vi "Gather_Deal_Data.vi"(8 "strModelChoice":string(combo)="WW6500", 10 "1号机端口":refnum<visa-resource-name>="COM1") -> (2 "缓冲区数据":u32=278, 3 "strResultArrayOut":string[](array[string])=["WaterLevel:22751", "WaterTemp:287", "AirTemp:300", "IPMTemp:300", "MotorActualRPM:0", "MotorTargetRPM:0", "FanActualRPM:0", "MemsSensorA:0", "MemsSensorB:35", "MemsSensorC:0", "WaterThermistorADC:33242", "TouchSensor:0", "LeakageSensor:0", "DCLink:321", "IsDoorOpen:0", "IsTimeShort:0", "Progress:0", "Step:0", "TotalRemainTime:3240", "StepRemainTime:0", "WeightSensingLowData:240", "WeightSensingResult:240", "ColdValve:0", "HotValve:0", "PreValve:0", "WaterShotValve:0", "BleachValve:0", "DryValve:0", "SteamValve:0", "SoftenerValve:0", "FilterValve:0", "IsDoorLocked:1", "SSRCommon:0", "MainRelay:1", "ACTUATOR2:0", "WaterDrainer:0", "CirculationPump:0", "WaterHeater:0", "DryHeater:0", "SteamHeater:0", "MotorDriveDirection:1", "IsDoubleDoorOpen:0", "IsDoubleDoorLock:1", "RunStateID:0", "PowerStateID:5", "SoundID:241", "ErrorCode:32323232", "OptionData:4112", "MainVersion:114494850", "SUBVersion:110484951", "InverterVersion:57484866", "MainVersion:32324853"], 9 "写指令":bool)   [LabVIEW 2011]
uses:
  <vilib>/Instr/_visa.llb/VISA Configure Serial Port (Instr).vi
  GlobalVariable/strGlobalVariable.vi
panel:
  out "mu083rdCmdSendCount":u8
  out "mu08SendCountStop":u8=9
  out "mbfSendStop":bool=TRUE
  out "WWorWD":bool
  out "1st_OnorOff":bool
  in  "chart":bool
  in  "Start":bool=TRUE
  out "mu08BufSize":u8=139
  out "mbfDealData":bool=TRUE
  in  "mu08SendCmd":u8=4
  in  "CmdNumCount":u8=76
  out "mu08ArrayBuf0":u8[](array[numeric])=[44, 7, 1, 44, 11, 0, 0, 12, 0, 0, 13, 0, 0, 21, 0, 0, 22, 0, 35, 23, 0, 0, 24, 129, 218, 29, 0, 0, 0, 0, 31, 0, 0, 33, 0, 34, 1, 65, 35, 0, 41, 0, 42, 0, 43, 0, 44, 12, 168, 45, 0, 0, 46, 0, 240, 47, 240, 48, 0, 49, 0, 50, 136, 51, 0, 52, 0, 53, 0, 54, 132, 58, 0, 59, 5, 60, 241, 61, 32, 32, 32, 32, 82, 4, 112, 83, 90, 3, 4, 0, 2, 4, 0, 0, 0, 0, 2, 0, 0, 0, 105, 201, 114, 49, 48, 50, 202, 110, 48, 49, 51, 203, 57, 48, 48, 66, 204, 32, 32, 48, 53, 251, 6, 239, 78, 90, 165, 139, 1, 240, 0, 1, 88, 223, 2, 1, 31, 3, 1, 44, 7, 1, 44, 11, 0, 0, 12, 0, 0, 13, 0, 0, 21, 0, 0, 22, 0, 35, 23, 0, 0, 24, 129, 218, 29, 0, 0, 0, 0, 31, 0, 0, 33, 0, 34, 1, 65, 35, 0, 41, 0, 42, 0, 43, 0, 44, 12, 168, 45, 0, 0, 46, 0, 240, 47, 240, 48, 0, 49, 0, 50, 136, 51, 0, 52, 0, 53, 0, 54, 132, 58, 0, 59, 5, 60, 241, 61, 32, 32, 32, 32, 82, 4, 112, 83, 90, 3, 4, 0, 2, 4, 0, 0, 0, 0, 2, 0, 0, 0, 105, 201, 114, 49, 48, 50, 202, 110, 48, 49, 51, 203, 57, 48, 48, 66, 204, 32, 32, 48, 53, 251, 6, 239, 78, 90, 165, 139, 1, 240, 0, 1, 88, 217, 2, 1, 31, 3, 1] format="0x%x"
  out "mu16ArrayBuf0":u16=278
  out "mu08ArrayDatas":u8[](array[numeric])=[90, 165, 139, 1, 240, 0, 1, 88, 223, 2, 1, 31, 3, 1, 44, 7, 1, 44, 11, 0, 0, 12, 0, 0, 13, 0, 0, 21, 0, 0, 22, 0, 35, 23, 0, 0, 24, 129, 218, 29, 0, 0, 0, 0, 31, 0, 0, 33, 0, 34, 1, 65, 35, 0, 41, 0, 42, 0, 43, 0, 44, 12, 168, 45, 0, 0, 46, 0, 240, 47, 240, 48, 0, 49, 0, 50, 136, 51, 0, 52, 0, 53, 0, 54, 132, 58, 0, 59, 5, 60, 241, 61, 32, 32, 32, 32, 82, 4, 112, 83, 90, 3, 4, 0, 2, 4, 0, 0, 0, 0, 2, 0, 0, 0, 105, 201, 114, 49, 48, 50, 202, 110, 48, 49, 51, 203, 57, 48, 48, 66, 204, 32, 32, 48, 53, 251, 6, 239, 78] format="0x%x"
  out "mu08ArrayDatasSize":u16=139
  out "命令":string
  in  "mbfUartClearOne":bool=TRUE
  out "Time":u32=400
  out "2nd_OnOrOff":bool
  in  "chart_2":bool
  in  "Start_2":bool
  in  "CmdNumCount 2":u8
  out "strResultArrayOut 2":string[](array[string])
  out "mbfDealData 2":bool
  out "mu08SendCmd_2":u8
  in  "写指令_2":bool=TRUE
  out "Time_2":u32=400
  out "缓冲区数据_2":u32=284
  out "mu08ArrayBuf0 2":u8[](array[numeric])=[90, 165, 142, 1, 240, 0, 1, 88, 200, 2, 0, 207, 3, 0, 219, 7, 1, 40, 11, 0, 0, 12, 0, 0, 13, 0, 0, 14, 0, 0, 21, 0, 0, 22, 0, 0, 23, 0, 0, 24, 150, 154, 29, 0, 0, 0, 0, 31, 0, 0, 33, 0, 34, 1, 64, 35, 0, 41, 0, 42, 0, 43, 0, 44, 12, 158, 45, 0, 0, 46, 0, 240, 47, 240, 48, 0, 49, 0, 50, 136, 51, 0, 52, 0, 53, 0, 54, 132, 58, 0, 59, 0, 60, 241, 61, 32, 32, 32, 32, 82, 64, 73, 83, 90, 2, 4, 0, 2, 4, 0, 0, 0, 0, 2, 0, 0, 0, 104, 201, 113, 49, 49, 53, 202, 70, 52, 48, 53, 203, 57, 48, 48, 66, 204, 32, 32, 48, 53, 251, 6, 87, 112, 90, 165, 142, 1, 240, 0, 1, 88, 200, 2, 0, 207, 3, 0, 219, 7, 1, 40, 11, 0, 0, 12, 0, 0, 13, 0, 0, 14, 0, 0, 21, 0, 0, 22, 0, 0, 23, 0, 0, 24, 150, 151, 29, 0, 0, 0, 0, 31, 0, 0, 33, 0, 34, 1, 64, 35, 0, 41, 0, 42, 0, 43, 0, 44, 12, 158, 45, 0, 0, 46, 0, 240, 47, 240, 48, 0, 49, 0, 50, 136, 51, 0, 52, 0, 53, 0, 54, 132, 58, 0, 59, 0, 60, 241, 61, 32, 32, 32, 32, 82, 64, 73, 83, 90, 2, 4, 0, 2, 4, 0, 0, 0, 0, 2, 0, 0, 0, 104, 201, 113, 49, 49, 53, 202, 70, 52, 48, 53, 203, 57, 48, 48, 66, 204, 32, 32, 48, 53, 251, 6, 95, 118] format="0x%x"
  out "mu16ArrayBuf0_2":u16=284
  out "mu08ArrayDatas_2":u8[](array[numeric])=[90, 165, 142, 1, 240, 0, 1, 88, 200, 2, 0, 207, 3, 0, 219, 7, 1, 40, 11, 0, 0, 12, 0, 0, 13, 0, 0, 14, 0, 0, 21, 0, 0, 22, 0, 0, 23, 0, 0, 24, 150, 154, 29, 0, 0, 0, 0, 31, 0, 0, 33, 0, 34, 1, 64, 35, 0, 41, 0, 42, 0, 43, 0, 44, 12, 158, 45, 0, 0, 46, 0, 240, 47, 240, 48, 0, 49, 0, 50, 136, 51, 0, 52, 0, 53, 0, 54, 132, 58, 0, 59, 0, 60, 241, 61, 32, 32, 32, 32, 82, 64, 73, 83, 90, 2, 4, 0, 2, 4, 0, 0, 0, 0, 2, 0, 0, 0, 104, 201, 113, 49, 49, 53, 202, 70, 52, 48, 53, 203, 57, 48, 48, 66, 204, 32, 32, 48, 53, 251, 6, 87, 112] format="0x%x"
  out "mu08ArrayDatasSize_2":u16=142
  out "mu08BufSize_2":u8
  in  "strModelChoice_2":string(combo)="WD5500"
  out "命令_2":string
  in  "mbfUartClearOne 2":bool=TRUE
  in  "2号机端口":refnum<visa-resource-name>="COM3"
  out "3rd_OnorOff":bool
  in  "chart_3":bool
  in  "Start_3":bool
  out "命令_3":string
  in  "CmdNumCount_3":u8
  out "mu16ArrayBuf0_3":u16=284
  out "mu08ArrayDatasSize_3":u16=142
  out "mu08BufSize_3":u8
  out "mu08ArrayBuf0_3":u8[](array[numeric])=[90, 165, 142, 1, 240, 0, 1, 88, 200, 2, 0, 207, 3, 0, 219, 7, 1, 40, 11, 0, 0, 12, 0, 0, 13, 0, 0, 14, 0, 0, 21, 0, 0, 22, 0, 0, 23, 0, 0, 24, 150, 154, 29, 0, 0, 0, 0, 31, 0, 0, 33, 0, 34, 1, 64, 35, 0, 41, 0, 42, 0, 43, 0, 44, 12, 158, 45, 0, 0, 46, 0, 240, 47, 240, 48, 0, 49, 0, 50, 136, 51, 0, 52, 0, 53, 0, 54, 132, 58, 0, 59, 0, 60, 241, 61, 32, 32, 32, 32, 82, 64, 73, 83, 90, 2, 4, 0, 2, 4, 0, 0, 0, 0, 2, 0, 0, 0, 104, 201, 113, 49, 49, 53, 202, 70, 52, 48, 53, 203, 57, 48, 48, 66, 204, 32, 32, 48, 53, 251, 6, 87, 112, 90, 165, 142, 1, 240, 0, 1, 88, 200, 2, 0, 207, 3, 0, 219, 7, 1, 40, 11, 0, 0, 12, 0, 0, 13, 0, 0, 14, 0, 0, 21, 0, 0, 22, 0, 0, 23, 0, 0, 24, 150, 151, 29, 0, 0, 0, 0, 31, 0, 0, 33, 0, 34, 1, 64, 35, 0, 41, 0, 42, 0, 43, 0, 44, 12, 158, 45, 0, 0, 46, 0, 240, 47, 240, 48, 0, 49, 0, 50, 136, 51, 0, 52, 0, 53, 0, 54, 132, 58, 0, 59, 0, 60, 241, 61, 32, 32, 32, 32, 82, 64, 73, 83, 90, 2, 4, 0, 2, 4, 0, 0, 0, 0, 2, 0, 0, 0, 104, 201, 113, 49, 49, 53, 202, 70, 52, 48, 53, 203, 57, 48, 48, 66, 204, 32, 32, 48, 53, 251, 6, 95, 118] format="0x%x"
  out "缓冲区数据_3":u32=284
  out "mu08ArrayDatas_3":u8[](array[numeric])=[90, 165, 142, 1, 240, 0, 1, 88, 200, 2, 0, 207, 3, 0, 219, 7, 1, 40, 11, 0, 0, 12, 0, 0, 13, 0, 0, 14, 0, 0, 21, 0, 0, 22, 0, 0, 23, 0, 0, 24, 150, 154, 29, 0, 0, 0, 0, 31, 0, 0, 33, 0, 34, 1, 64, 35, 0, 41, 0, 42, 0, 43, 0, 44, 12, 158, 45, 0, 0, 46, 0, 240, 47, 240, 48, 0, 49, 0, 50, 136, 51, 0, 52, 0, 53, 0, 54, 132, 58, 0, 59, 0, 60, 241, 61, 32, 32, 32, 32, 82, 64, 73, 83, 90, 2, 4, 0, 2, 4, 0, 0, 0, 0, 2, 0, 0, 0, 104, 201, 113, 49, 49, 53, 202, 70, 52, 48, 53, 203, 57, 48, 48, 66, 204, 32, 32, 48, 53, 251, 6, 87, 112] format="0x%x"
  in  "strModelChoice 2":string(combo)="WD5500"
  in  "写指令_3":bool=TRUE
  in  "3号机端口":refnum<visa-resource-name>="COM3"
  in  "mbfUartClearOne_3":bool=TRUE
  out "mbfDealData_3":bool
  out "Time_3":u32=400
  out "strResultArrayOut_3":string[](array[string])
  out "mu08SendCmd_2 2":u8
  out "4ed_OronOff":bool
  in  "chart_4":bool
  in  "Start_4":bool
  in  "strModelChoice_4":string(combo)="WD5500"
  out "Time_4":u32=400
  out "mbfDealData_4":bool
  in  "mbfUartClearOne_4":bool=TRUE
  out "strResultArrayOut_4":string[](array[string])
  out "mu08SendCmd_4":u8
  out "命令_4":string
  in  "写指令_4":bool=TRUE
  out "mu08ArrayDatas_4":u8[](array[numeric])=[90, 165, 142, 1, 240, 0, 1, 88, 200, 2, 0, 207, 3, 0, 219, 7, 1, 40, 11, 0, 0, 12, 0, 0, 13, 0, 0, 14, 0, 0, 21, 0, 0, 22, 0, 0, 23, 0, 0, 24, 150, 154, 29, 0, 0, 0, 0, 31, 0, 0, 33, 0, 34, 1, 64, 35, 0, 41, 0, 42, 0, 43, 0, 44, 12, 158, 45, 0, 0, 46, 0, 240, 47, 240, 48, 0, 49, 0, 50, 136, 51, 0, 52, 0, 53, 0, 54, 132, 58, 0, 59, 0, 60, 241, 61, 32, 32, 32, 32, 82, 64, 73, 83, 90, 2, 4, 0, 2, 4, 0, 0, 0, 0, 2, 0, 0, 0, 104, 201, 113, 49, 49, 53, 202, 70, 52, 48, 53, 203, 57, 48, 48, 66, 204, 32, 32, 48, 53, 251, 6, 87, 112] format="0x%x"
  in  "CmdNumCount_4":u8
  out "缓冲区数据_4":u32=284
  out "mu08BufSize_4":u8
  out "mu08ArrayBuf0_4":u8[](array[numeric])=[90, 165, 142, 1, 240, 0, 1, 88, 200, 2, 0, 207, 3, 0, 219, 7, 1, 40, 11, 0, 0, 12, 0, 0, 13, 0, 0, 14, 0, 0, 21, 0, 0, 22, 0, 0, 23, 0, 0, 24, 150, 154, 29, 0, 0, 0, 0, 31, 0, 0, 33, 0, 34, 1, 64, 35, 0, 41, 0, 42, 0, 43, 0, 44, 12, 158, 45, 0, 0, 46, 0, 240, 47, 240, 48, 0, 49, 0, 50, 136, 51, 0, 52, 0, 53, 0, 54, 132, 58, 0, 59, 0, 60, 241, 61, 32, 32, 32, 32, 82, 64, 73, 83, 90, 2, 4, 0, 2, 4, 0, 0, 0, 0, 2, 0, 0, 0, 104, 201, 113, 49, 49, 53, 202, 70, 52, 48, 53, 203, 57, 48, 48, 66, 204, 32, 32, 48, 53, 251, 6, 87, 112, 90, 165, 142, 1, 240, 0, 1, 88, 200, 2, 0, 207, 3, 0, 219, 7, 1, 40, 11, 0, 0, 12, 0, 0, 13, 0, 0, 14, 0, 0, 21, 0, 0, 22, 0, 0, 23, 0, 0, 24, 150, 151, 29, 0, 0, 0, 0, 31, 0, 0, 33, 0, 34, 1, 64, 35, 0, 41, 0, 42, 0, 43, 0, 44, 12, 158, 45, 0, 0, 46, 0, 240, 47, 240, 48, 0, 49, 0, 50, 136, 51, 0, 52, 0, 53, 0, 54, 132, 58, 0, 59, 0, 60, 241, 61, 32, 32, 32, 32, 82, 64, 73, 83, 90, 2, 4, 0, 2, 4, 0, 0, 0, 0, 2, 0, 0, 0, 104, 201, 113, 49, 49, 53, 202, 70, 52, 48, 53, 203, 57, 48, 48, 66, 204, 32, 32, 48, 53, 251, 6, 95, 118] format="0x%x"
  in  "4号机端口":refnum<visa-resource-name>="COM3"
  out "mu08ArrayDatasSize_4":u16=142
  out "mu16ArrayBuf0_4":u16=284
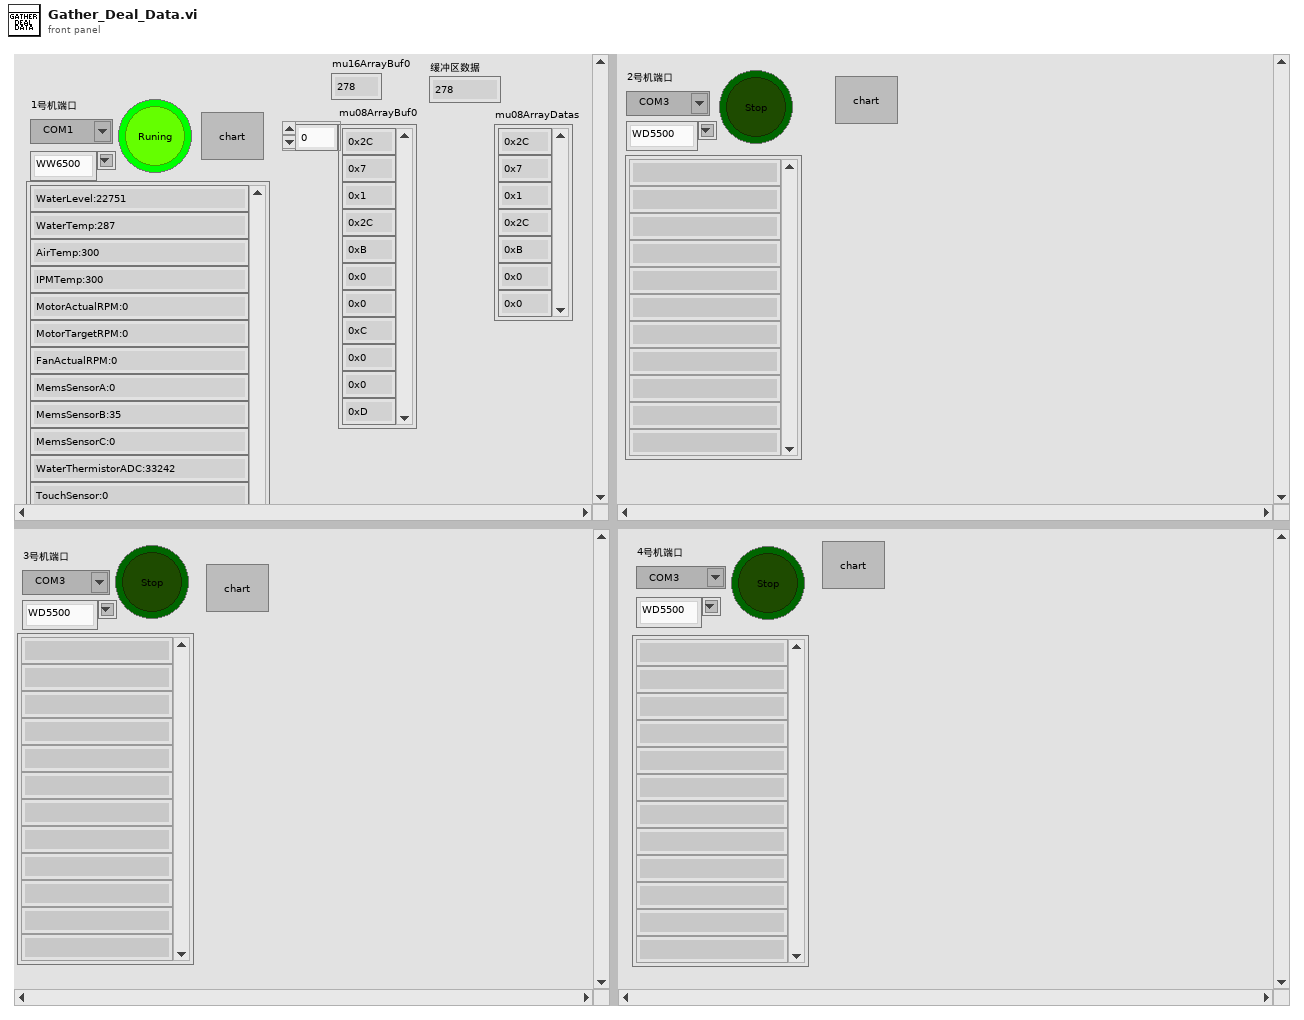
[diagram p1: front panel]
types:
  T1 = enum16{"open", "replace", "create", "open or create", "replace or create", "replace or create with confirmation"}
  T2 = enum32{"Invalid", "Standard", "Closed", "Hidden", "Minimized", "Maximized"}
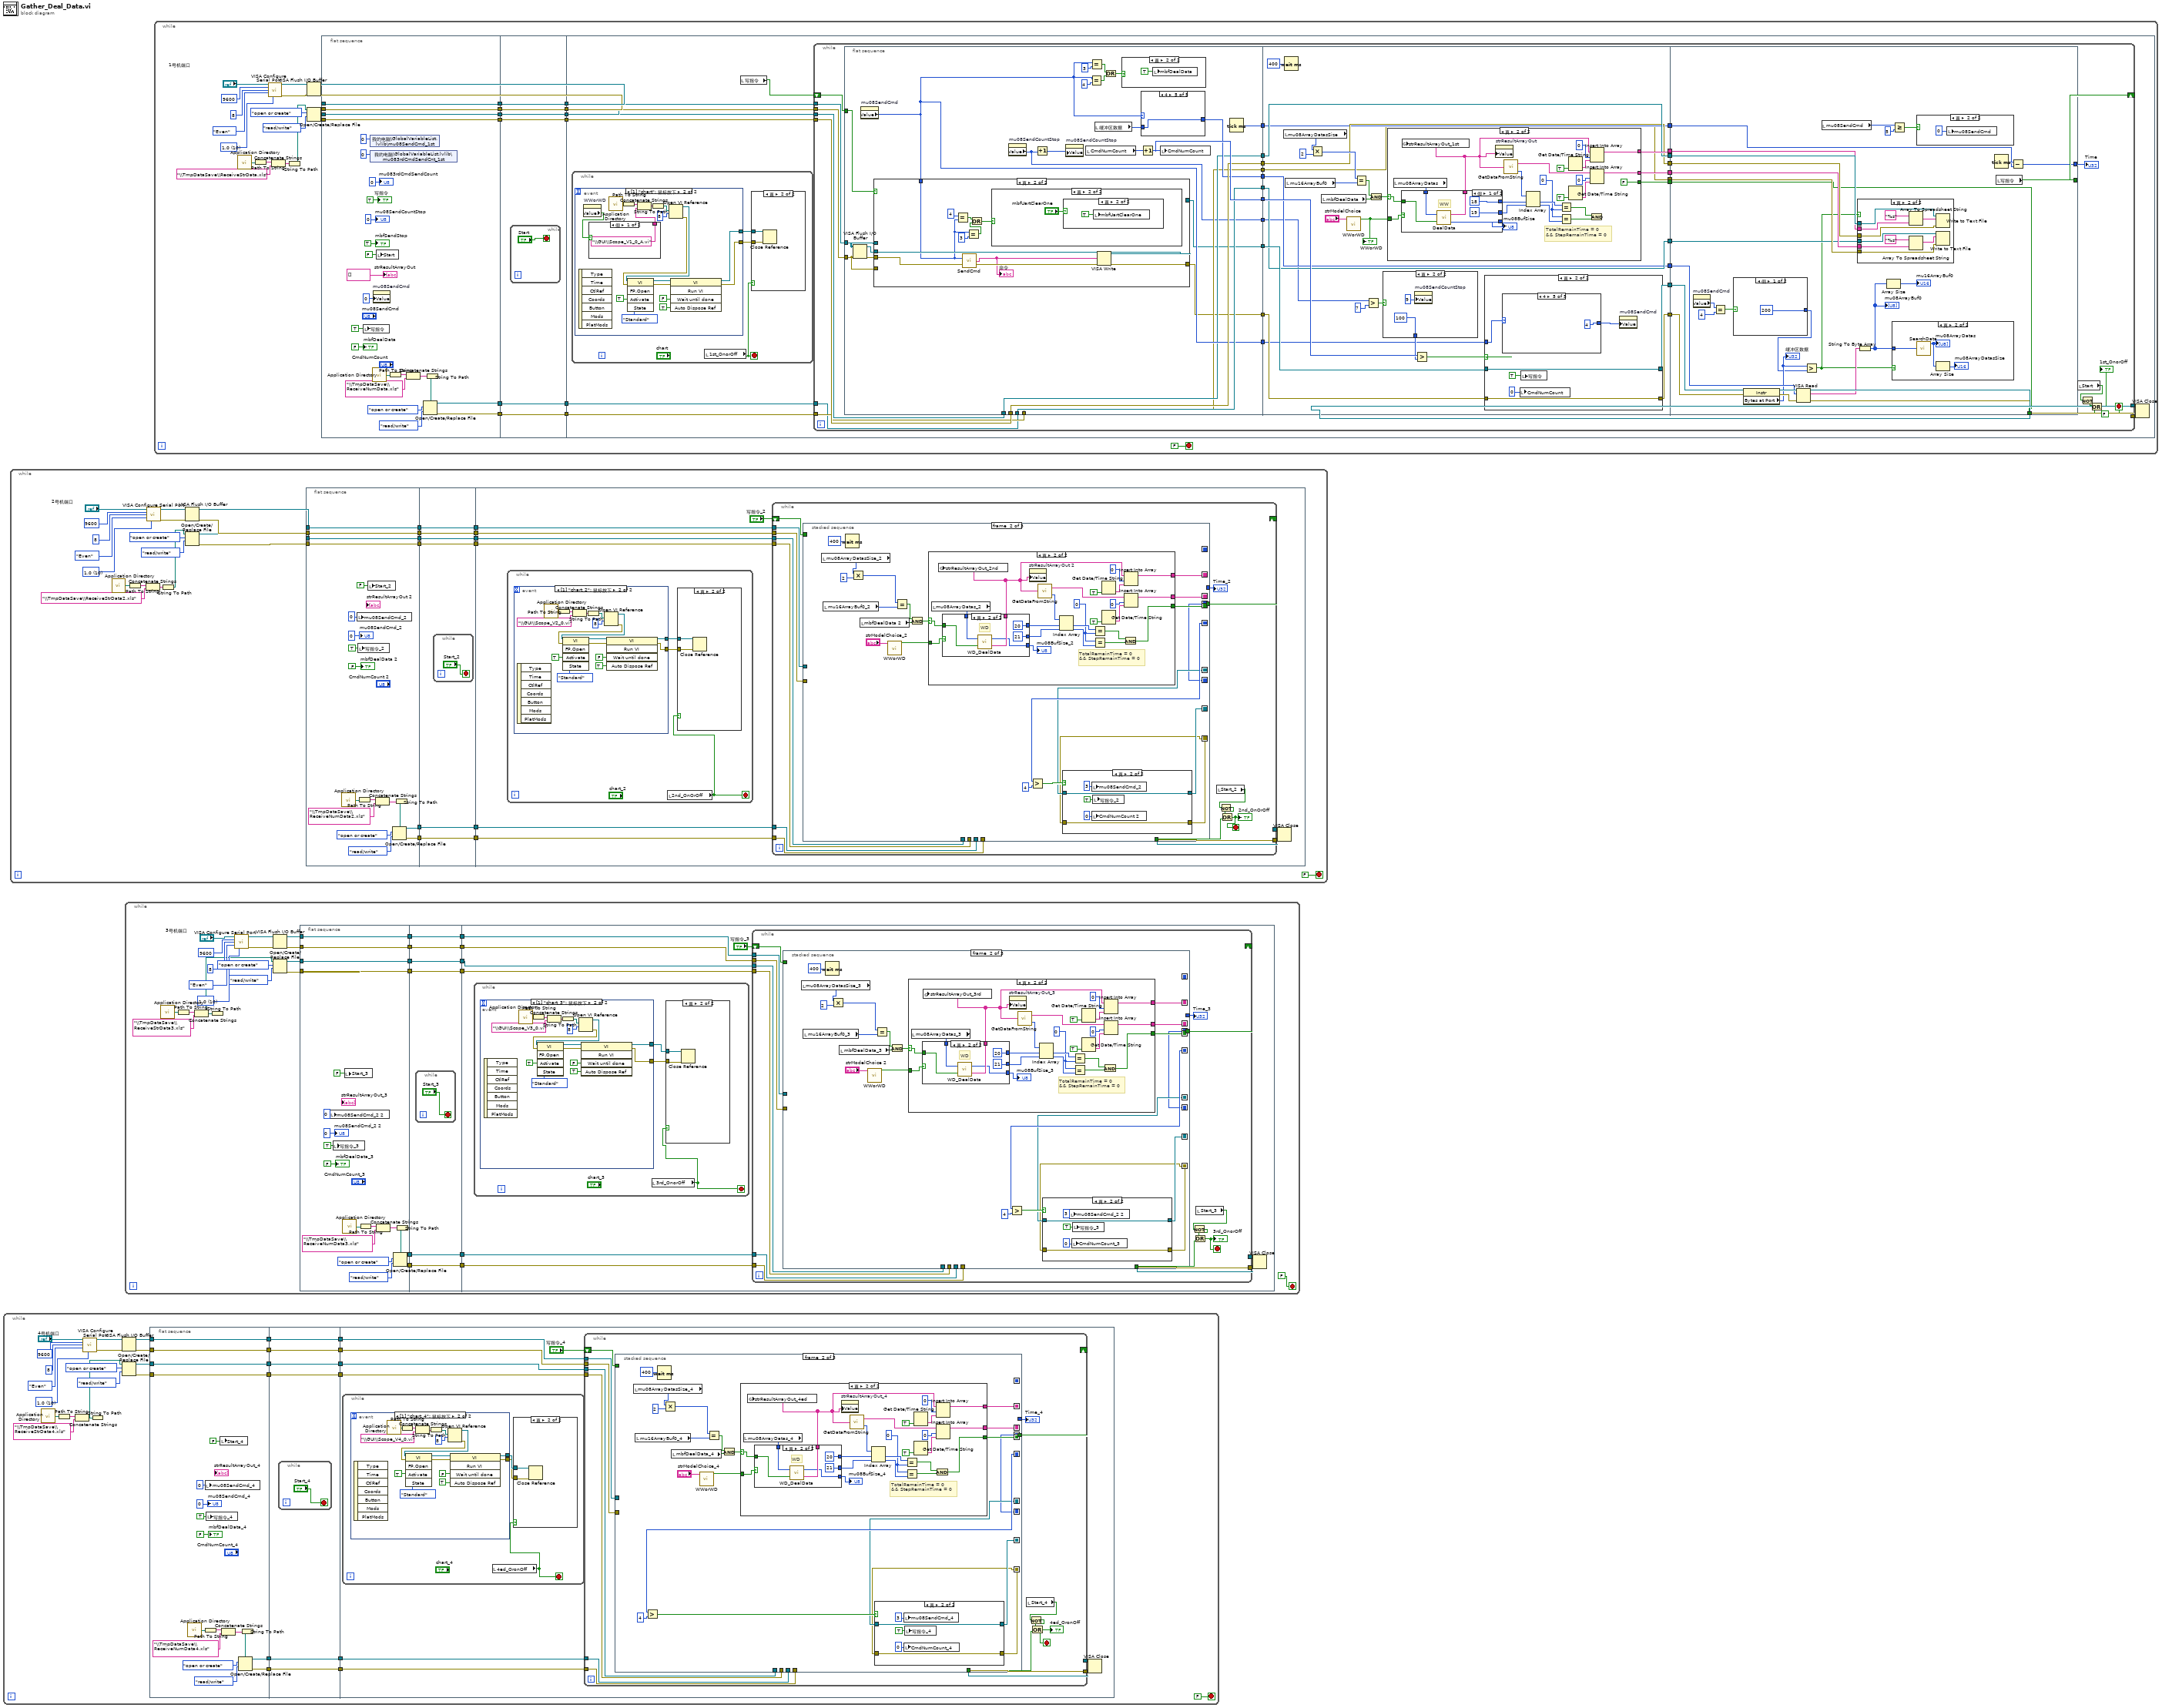
[diagram p0: block diagram]
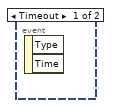
[diagram p3: hidden frame]
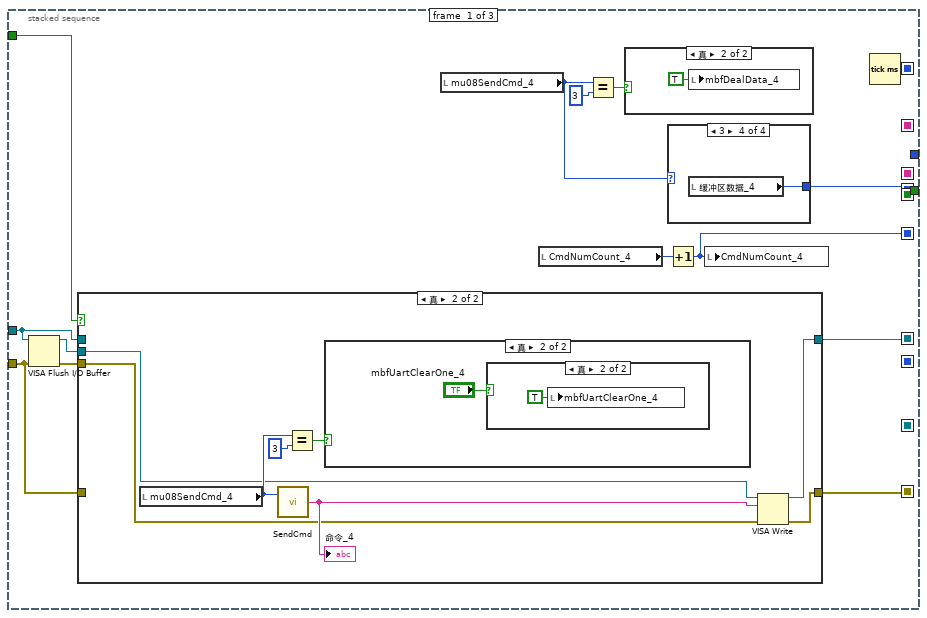
[diagram p4: hidden frame]
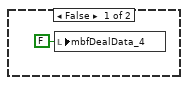
[diagram p5: hidden frame]
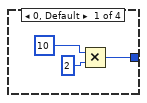
[diagram p6: hidden frame]
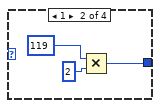
[diagram p7: hidden frame]
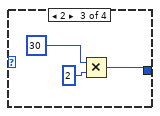
[diagram p8: hidden frame]
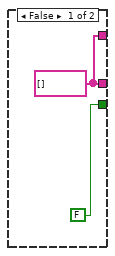
[diagram p12: hidden frame]
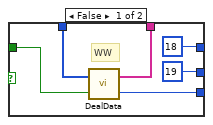
[diagram p13: hidden frame]
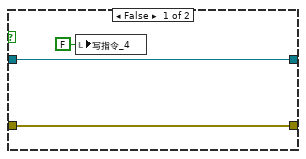
[diagram p14: hidden frame]
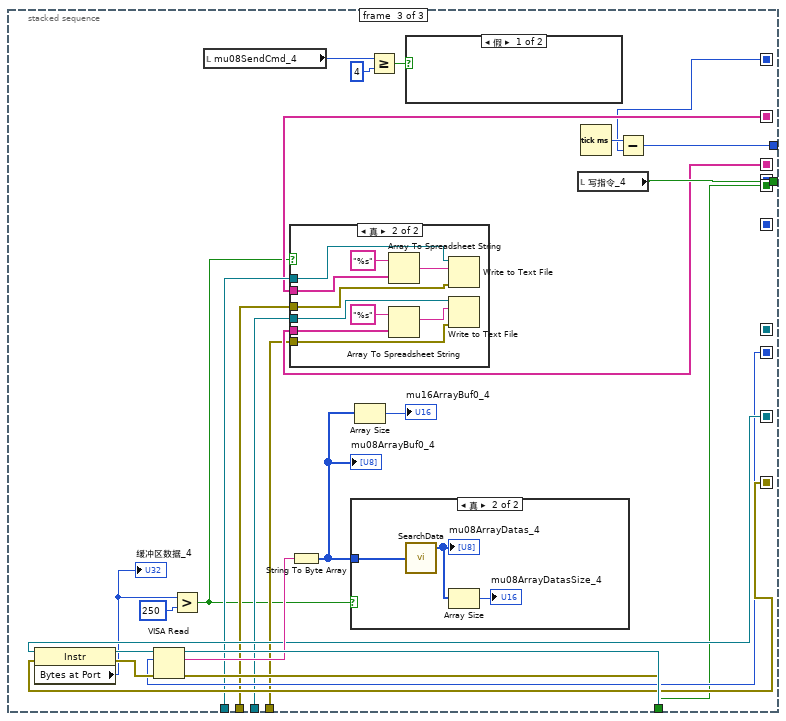
[diagram p15: hidden frame]
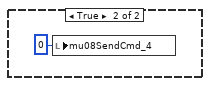
[diagram p18: hidden frame]
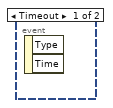
[diagram p20: hidden frame]
diagram:
  n1 = while {
    stop <- FALSE stop-if-true
    w15 = u16 10 items=["1.0"=10, "1.5"=15, "2.0"=20] ("stop bits (10: 1 bit)")
    n2 = call <vilib>:"Application Directory.vi"() -> ("Application Directory"=w5:path)
    n3 = Path To String(path=w5) -> (string=w4:string)
    n4 = Concatenate Strings(w4, "\\TmpDataSave\\ReceiveStrData4.xls" ("字符串")) -> (w2:string)
    n5 = call-poly "VISA Configure Serial Port"("VISA resource name"="4号机端口", "baud rate (9600)"=u32 9600, "data bits (8)"=u16 8, "parity (0:none)"=enum16{"None", "Odd", "Even", "Mark", "Space"}."Even", "stop bits (10: 1 bit)"=w15) -> ("VISA resource name out"=w14:refnum<visa-resource-name>, "error out"=w13:errorcluster)  [unwired: 9 in]
    n6 = String To Path(string=w2) -> (path=w8:path)
    n7 = VISA Flush I/O Buffer(VISA resource name=w14, error in (no error)=w13) -> (VISA resource name out=w12:refnum<visa-resource-name>, error out=w11:errorcluster)  [unwired: 1 in]
    n8 = Open/Create/Replace File(file path (use dialog)=w8, operation (0:open)=T1."open or create" ("操作(0:open)"), access (0:read/write)=enum16{"read/write", "read-only", "write-only"}."read/write" ("权限(0:read/write)")) -> (refnum out=w7:refnum<file>, error out=w6:errorcluster)  [unwired: 3 in, 1 out]
    n9 = flat-sequence {
      tunnel: w6 -> [w46]
      tunnel: w7 -> [w47]
      tunnel: w11 -> [w48]
      tunnel: w12 -> [w49]
      tunnel: [w49] -> w31
      tunnel: [w48] -> w30
      tunnel: [w47] -> w29
      tunnel: [w46] -> w28
      tunnel: [w32] -> w27
      tunnel: [w33] -> w26
      tunnel: [w55] -> w25
      tunnel: [w54] -> w24
      tunnel: [w53] -> w23
      tunnel: [w52] -> w22
      tunnel: [w51] -> w21
      tunnel: [w50] -> w20
      tunnel: w31 -> [w55]
      tunnel: w30 -> [w54]
      tunnel: w29 -> [w53]
      tunnel: w28 -> [w52]
      tunnel: w27 -> [w51]
      tunnel: w26 -> [w50]
      tunnel: w25 -> [w62]
      tunnel: w24 -> [w61]
      tunnel: w23 -> [w60]
      tunnel: w22 -> [w59]
      tunnel: w21 -> [w58]
      tunnel: w20 -> [w57]
      frame #0 {
        n10 = call <vilib>:"Application Directory.vi"() -> ("Application Directory"=w37:path)
        n11 = Path To String(path=w37) -> (string=w38:string)
        n12 = local write "mu08SendCmd_4"(u8 0 ("Cmd值")) -> ()
        n13 = local write "写指令_4"(TRUE ("写指令")) -> ()
        n14 = local write "Start_4"(FALSE ("Start_4")) -> ()
        n15 = Concatenate Strings(w38, "\\TmpDataSave\\ReceiveNumData4.xls" ("字符串")) -> (w40:string)
        n16 = String To Path(string=w40) -> (path=w36:path)
        n17 = Open/Create/Replace File(file path (use dialog)=w36, operation (0:open)=T1."open or create" ("操作(0:open)"), access (0:read/write)=enum16{"read/write", "read-only", "write-only"}."read/write" ("权限(0:read/write)")) -> (refnum out=w33:refnum<file>, error out=w32:errorcluster)  [unwired: 3 in, 1 out]
        "mu08SendCmd_4" <- u8 0 ("mu08SendCmd")
        "mbfDealData_4" <- FALSE ("mbfDealData")
      }
      frame #1 {
        n18 = while {
          stop <- "Start_4" stop-if-true
        }
      }
      frame #2 {
        n19 = while {
          stop <- w67 stop-if-true
          n20 = event shown="[1] \"chart_4\": 鼠标按下" {
            selector: _ -> [_ _]
            dyn-events: _ -> [_ _]
            timeout: _ -> [_ _]
            tunnel: [_ w72] -> w68
            tunnel: [_ w71] -> w66
            event Timeout {
              n21 = event-data() -> ()  [unwired: 1 in, 2 out]
            }
            event "chart_4": Mouse Down {
              n22 = event-data() -> ()  [unwired: 1 in, 7 out]
              n23 = call <vilib>:"Application Directory.vi"() -> ("Application Directory"=w84:path)
              n24 = Path To String(path=w84) -> (string=w83:string)
              n25 = Concatenate Strings(w83, "\\GUI\\Scope_V4_0.vi" ("名称或相对路径")) -> (w81:string)
              n26 = String To Path(string=w81) -> (path=w85:path)
              n27 = Open VI Reference(vi path=w85, options=8 ("选项")) -> (vi reference=w80:refnum<vi>, error out=w79:errorcluster)  [unwired: 4 in]
              n28 = invoke class="VI" method="FP.Open"(reference=w80, error in=w79, "Activate"=TRUE ("激活？"), "State"=T2."Standard" ("州")) -> (reference out=w76:refnum<vi>, error out=w75:errorcluster)  [unwired: 1 in, 3 out]
              n29 = invoke class="VI" method="Run VI"(reference=w76, error in=w75, "Wait until done"=FALSE ("结束前等待"), "Auto Dispose Ref"=TRUE ("自动销毁引用")) -> (reference out=w72:refnum<vi>, error out=w71:errorcluster)  [unwired: 1 in, 3 out]
            }
          }
          n30 = local read "4ed_OronOff"() -> (w67:bool)
          n31 = case shown="真" w67 {
            tunnel: w68 -> [_ w69]
            tunnel: w66 -> [_ w70]
            frame False {
            }
            frame True {
              n32 = Close Reference(reference=w69, error in (no error)=w70) -> ()  [unwired: 1 out]
            }
          }
        }
        n33 = while {
          tunnel: w62 -> [w101]
          tunnel: w61 -> [w100]
          tunnel: [w99] -> w65
          tunnel: [w98] -> w64
          shift-right: [w96] -> _
          shift-left: "写指令_4" -> [w97]
          tunnel: w60 -> [w95]
          tunnel: w59 -> [w94]
          tunnel: w58 -> [w92]
          tunnel: w57 -> [w91]
          stop <- w88 stop-if-true
          n34 = stacked-sequence {
            seq-local: [w115 _ _] -> [_ w155 _]
            seq-local: [w114 _ _] -> [_ w154 _]
            seq-local: [w111 _ _] -> [_ w158 _]
            seq-local: [w102 _ _] -> [_ w142 _]
            seq-local: [w103 _ _] -> [_ w152 _]
            seq-local: [_ w157 _] -> [_ _ w228]
            seq-local: [_ w156 _] -> [_ _ w227]
            seq-local: [_ w153 _] -> [_ _ w218]
            seq-local: [_ w152 _] -> [_ _ w216]
            seq-local: [_ w151 _] -> [_ _ w214]
            seq-local: [_ w146 _] -> [_ _ w207]
            seq-local: [_ w142 _] -> [_ _ w223]
            tunnel: w101 -> [w107 _ _]
            tunnel: w100 -> [w106 _ _]
            tunnel: w97 -> [w113 _ _]
            tunnel: [_ _ w231] -> w99
            tunnel: [_ _ w230] -> w98
            tunnel: [_ _ w222] -> w96
            tunnel: w95 -> [_ _ w220]
            tunnel: w94 -> [_ _ w219]
            tunnel: [_ _ w215] -> w93
            tunnel: w92 -> [_ _ w213]
            tunnel: w91 -> [_ _ w212]
            tunnel: [_ _ w207] -> w87
            frame #0 {
              n35 = VISA Flush I/O Buffer(VISA resource name=w107, error in (no error)=w106) -> (VISA resource name out=w104:refnum<visa-resource-name>, error out=w105:errorcluster)  [unwired: 1 in]
              n36 = case shown="真" w113 {
                tunnel: w107 -> [w129 _]
                tunnel: w106 -> [w128 _]
                tunnel: [w129 w137] -> w115
                tunnel: [w128 w136] -> w114
                tunnel: w105 -> [_ w131]
                tunnel: w104 -> [_ w130]
                frame False {
                }
                frame True {
                  n37 = local read "mu08SendCmd_4"() -> (w133:u8)
                  n38 = call "SendCmd.vi"("索引 (行)"=w133) -> ("字符串"=w135:string)  [unwired: 1 in]
                  "命令_4" <- w135
                  n39 = Equal?(x=w133, y=u8 3) -> (x = y?=w132:bool)
                  n40 = case shown="真" w132 {
                    frame False {
                    }
                    frame True {
                      n41 = case shown="真" "mbfUartClearOne_4" {
                        frame False {
                        }
                        frame True {
                          n42 = local write "mbfUartClearOne_4"(TRUE ("mbfUartClearOne")) -> ()
                        }
                      }
                    }
                  }
                  n43 = VISA Write(VISA resource name=w130, write buffer=w135, error in (no error)=w131) -> (VISA resource name out=w137:refnum<visa-resource-name>, error out=w136:errorcluster)  [unwired: 1 out]
                }
              }
              n44 = local read "mu08SendCmd_4"() -> (w110:u8)
              n45 = local read "CmdNumCount_4"() -> (w112:u8)
              n46 = Equal?(x=w110, y=u8 3) -> (x = y?=w108:bool)
              n47 = case shown="真" w108 {
                frame False {
                  n48 = local write "mbfDealData_4"(FALSE ("mbfDealData")) -> ()
                }
                frame True {
                  n49 = local write "mbfDealData_4"(TRUE ("mbfDealData")) -> ()
                }
              }
              n50 = case shown="3" w110 {
                tunnel: [w118 w121 w124 w127] -> w102
                frame 0, Default {
                  n51 = Multiply(x=10, y=2) -> (x*y=w118:i32)
                }
                frame 1 {
                  n52 = Multiply(x=119, y=2) -> (x*y=w121:i32)
                }
                frame 2 {
                  n53 = Multiply(x=30, y=2) -> (x*y=w124:i32)
                }
                frame 3 {
                  n54 = local read "缓冲区数据_4"() -> (w127:u32)
                }
              }
              n55 = Increment(x=w112) -> (x+1=w111:u8)
              n56 = local write "CmdNumCount_4"(w111) -> ()
              n57 = Tick Count (ms)() -> (millisecond timer value=w103:u32)
            }
            frame #1 {
              n58 = local read "mu08ArrayDatasSize_4"() -> (w145:u16)
              n59 = local read "mu16ArrayBuf0_4"() -> (w150:u16)
              n60 = Greater?(x=w158, y=u8 4) -> (0:w159:bool)
              n61 = Wait (ms)(milliseconds to wait=u32 400 ("等待时间（毫秒）")) -> ()  [unwired: 1 out]
              n62 = Multiply(x=w145, y=u8 2) -> (x*y=w143:u16)
              n63 = local read "mbfDealData_4"() -> (w149:bool)
              n64 = call "WWorWD.vi"("strModelChoice"="strModelChoice_4") -> ("WWorWD"=w140:bool)  [unwired: 9 in, 1 out]
              n65 = Equal?(x=w143, y=w150) -> (x = y?=w148:bool)
              n66 = And(x=w148, y=w149) -> (x .and. y?=w147:bool)
              n67 = case shown="真" w147 {
                selector: w147 -> [_ w166]
                tunnel: [w163 w184] -> w153
                tunnel: [w163 w179] -> w151
                tunnel: [FALSE w171] -> w146
                tunnel: w140 -> [_ w167]
                frame False {
                  w163 = string[] []
                }
                frame True {
                  w175 = u32 0 ("y")
                  # "TotalRemainTime = 0\n&& StepRemainTime = 0"
                  n68 = local read "mu08ArrayDatas_4"() -> (w170:u8[])
                  n69 = case shown="真" w167 {
                    tunnel: [w192 w198] -> w164
                    tunnel: [w191 w197] -> w165
                    tunnel: w170 -> [w190 w196]
                    tunnel: [18 ("索引") 20 ("索引")] -> w169
                    tunnel: [19 ("索引") 21 ("索引")] -> w168
                    tunnel: w166 -> [w187 w193]
                    frame False {
                      # "WW"
                      n70 = call "DealData.vi"("mbfDealData"=w187, "ArrayIn"=w190) -> ("mu08BufSize"=w191:u8, "Result"=w192:string[])
                    }
                    frame True {
                      # "WD"
                      n71 = call "WD_DealData.vi"("mbfDealData"=w193, "ArrayIn"=w196) -> ("ResultArrayOut"=w198:string[], "mu08BufSize"=w197:u8)
                    }
                  }
                  "mu08BufSize_4" <- w165
                  n72 = global write "strGlobalVariable.vi" "strResultArrayOut_4ed"(w164) -> ()
                  n73 = property on="strResultArrayOut_4" class="Arr (严格)"("Value"=w164) -> ()  [unwired: 2 in, 2 out]
                  n74 = call "GetDataFromString.vi"("strArrayIn"=w164) -> ("strArrayBuf"=w178:string[], "mu32ArrayOut"=w177:u32[])
                  n75 = Index Array(array=w177, index #1=w169, index #2=w168) -> (element #1=w176:u32, element #2=w174:u32)
                  n76 = Equal?(x=w176, y=w175) -> (x = y?=w173:bool)
                  n77 = Equal?(x=w175, y=w174) -> (x = y?=w172:bool)
                  n78 = Get Date/Time String(want seconds? (F)=TRUE ("需要秒？(F)")) -> (time string=w185:string)  [unwired: 2 in, 1 out]
                  n79 = Get Date/Time String(want seconds? (F)=TRUE ("需要秒？(F)")) -> (time string=w181:string)  [unwired: 2 in, 1 out]
                  n80 = And(x=w173, y=w172) -> (x .and. y?=w171:bool)
                  n81 = Insert Into Array(array=w164, index=0 ("索引"), new element=w185) -> (w184:string[])
                  n82 = Insert Into Array(array=w178, index=0 ("索引"), new element=w181) -> (w179:string[])
                }
              }
              n83 = case shown="真" w159 {
                tunnel: [w200 w204] -> w157
                tunnel: [w199 w203] -> w156
                tunnel: w155 -> [w200 w204]
                tunnel: w154 -> [w199 w203]
                frame False {
                  n84 = local write "写指令_4"(FALSE ("写指令")) -> ()
                }
                frame True {
                  n85 = local write "mu08SendCmd_4"(u8 3 ("mu08SendCmd")) -> ()
                  n86 = local write "CmdNumCount_4"(u8 0 ("CmdNumCount")) -> ()
                  n87 = local write "写指令_4"(TRUE ("写指令")) -> ()
                }
              }
            }
            frame #2 {
              n88 = property class="Instr"(reference=w228, error in=w227) -> (reference out=w233:refnum<visa-resource-name>, error out=w232:errorcluster, "Bytes at Port"=w210:u32)
              "缓冲区数据_4" <- w210
              n89 = VISA Read(VISA resource name=w233, byte count=w223, error in (no error)=w232) -> (VISA resource name out=w231:refnum<visa-resource-name>, read buffer=w229:string, error out=w230:errorcluster)  [unwired: 1 out]
              n90 = Greater?(x=w210, y=250) -> (0:w209:bool)
              n91 = local read "mu08SendCmd_4"() -> (w226:u8)
              n92 = case shown="真" w209 {
                tunnel: w220 -> [_ w244]
                tunnel: w219 -> [_ w243]
                tunnel: w218 -> [_ w242]
                tunnel: w214 -> [_ w241]
                tunnel: w213 -> [_ w238]
                tunnel: w212 -> [_ w237]
                frame False {
                }
                frame True {
                  n93 = Array To Spreadsheet String(array=w242, 3:"%s" ("格式字符串")) -> (spreadsheet string=w246:string)  [unwired: 1 in]
                  n94 = Array To Spreadsheet String(array=w241, 3:"%s" ("格式字符串")) -> (spreadsheet string=w239:string)  [unwired: 1 in]
                  n95 = Write to Text File(file (use dialog)=w244, text=w246, error in=w243) -> ()  [unwired: 1 in, 3 out]
                  n96 = Write to Text File(file (use dialog)=w237, text=w239, error in=w238) -> ()  [unwired: 1 in, 3 out]
                }
              }
              n97 = String To Byte Array(string=w229) -> (unsigned byte array=w208:u8[])
              "mu08ArrayBuf0_4" <- w208
              n98 = case shown="真" w209 {
                tunnel: w208 -> [_ w235]
                frame False {
                }
                frame True {
                  n99 = call "SearchData.vi"("ArrayIn"=w235) -> ("ArrayOut"=w234:u8[])  [unwired: 2 out]
                  "mu08ArrayDatas_4" <- w234
                  n100 = Array Size(array=w234) -> (size(s)=→"mu08ArrayDatasSize_4":i32)
                }
              }
              n101 = Array Size(array=w208) -> (size(s)=→"mu16ArrayBuf0_4":i32)
              n102 = Greater Or Equal?(x=w226, y=u8 4) -> (x >= y?=w224:bool)
              n103 = case shown="假" w224 {
                frame False {
                }
                frame True {
                  n104 = local write "mu08SendCmd_4"(u8 0 ("Cmd值")) -> ()
                }
              }
              n105 = local read "写指令_4"() -> (w222:bool)
              n106 = Tick Count (ms)() -> (millisecond timer value=w217:u32)
              n107 = Subtract(x=w217, y=w216) -> (x-y=w215:u32)
            }
          }
          "Time_4" <- w93
          n108 = local read "Start_4"() -> (w90:bool)
          n109 = Not(x=w90) -> (.not. x?=w89:bool)
          n110 = Or(x=w89, y=w87) -> (x .or. y?=w88:bool)
          "4ed_OronOff" <- w88
        }
        n111 = VISA Close(VISA resource name=w65, error in (no error)=w64) -> ()  [unwired: 1 out]
      }
    }
  }
  n112 = while {
    stop <- FALSE stop-if-true
    w262 = u16 10 items=["1.0"=10, "1.5"=15, "2.0"=20] ("stop bits (10: 1 bit)")
    n113 = call <vilib>:"Application Directory.vi"() -> ("Application Directory"=w252:path)
    n114 = Path To String(path=w252) -> (string=w251:string)
    n115 = Concatenate Strings(w251, "\\TmpDataSave\\ReceiveStrData2.xls" ("字符串")) -> (w249:string)
    n116 = call-poly "VISA Configure Serial Port"("VISA resource name"="2号机端口", "baud rate (9600)"=u32 9600, "data bits (8)"=u16 8, "parity (0:none)"=enum16{"None", "Odd", "Even", "Mark", "Space"}."Even", "stop bits (10: 1 bit)"=w262) -> ("VISA resource name out"=w261:refnum<visa-resource-name>, "error out"=w260:errorcluster)  [unwired: 9 in]
    n117 = String To Path(string=w249) -> (path=w255:path)
    n118 = VISA Flush I/O Buffer(VISA resource name=w261, error in (no error)=w260) -> (VISA resource name out=w259:refnum<visa-resource-name>, error out=w258:errorcluster)  [unwired: 1 in]
    n119 = Open/Create/Replace File(file path (use dialog)=w255, operation (0:open)=T1."open or create" ("操作(0:open)"), access (0:read/write)=enum16{"read/write", "read-only", "write-only"}."read/write" ("权限(0:read/write)")) -> (refnum out=w254:refnum<file>, error out=w253:errorcluster)  [unwired: 3 in, 1 out]
    n120 = flat-sequence {
      tunnel: w253 -> [w293]
      tunnel: w254 -> [w294]
      tunnel: w258 -> [w295]
      tunnel: w259 -> [w296]
      tunnel: [w296] -> w278
      tunnel: [w295] -> w277
      tunnel: [w294] -> w276
      tunnel: [w293] -> w275
      tunnel: [w280] -> w274
      tunnel: [w279] -> w273
      tunnel: [w302] -> w272
      tunnel: [w301] -> w271
      tunnel: [w300] -> w270
      tunnel: [w299] -> w269
      tunnel: [w298] -> w268
      tunnel: [w297] -> w267
      tunnel: w278 -> [w302]
      tunnel: w277 -> [w301]
      tunnel: w276 -> [w300]
      tunnel: w275 -> [w299]
      tunnel: w274 -> [w297]
      tunnel: w273 -> [w298]
      tunnel: w272 -> [w309]
      tunnel: w271 -> [w308]
      tunnel: w270 -> [w307]
      tunnel: w269 -> [w306]
      tunnel: w268 -> [w305]
      tunnel: w267 -> [w304]
      frame #0 {
        n121 = call <vilib>:"Application Directory.vi"() -> ("Application Directory"=w284:path)
        n122 = local write "mu08SendCmd_2"(u8 0 ("Cmd值")) -> ()
        n123 = local write "写指令_2"(TRUE ("写指令")) -> ()
        n124 = Path To String(path=w284) -> (string=w285:string)
        n125 = local write "Start_2"(FALSE ("Start_2")) -> ()
        n126 = Concatenate Strings(w285, "\\TmpDataSave\\ReceiveNumData2.xls" ("字符串")) -> (w287:string)
        n127 = String To Path(string=w287) -> (path=w283:path)
        n128 = Open/Create/Replace File(file path (use dialog)=w283, operation (0:open)=T1."open or create" ("操作(0:open)"), access (0:read/write)=enum16{"read/write", "read-only", "write-only"}."read/write" ("权限(0:read/write)")) -> (refnum out=w280:refnum<file>, error out=w279:errorcluster)  [unwired: 3 in, 1 out]
        "mu08SendCmd_2" <- u8 0 ("mu08SendCmd")
        "mbfDealData 2" <- FALSE ("mbfDealData")
      }
      frame #1 {
        n129 = while {
          stop <- "Start_2" stop-if-true
        }
      }
      frame #2 {
        n130 = while {
          stop <- w315 stop-if-true
          n131 = event shown="[1] \"chart_2\": 鼠标按下" {
            selector: _ -> [_ _]
            dyn-events: _ -> [_ _]
            timeout: _ -> [_ _]
            tunnel: [_ w319] -> w314
            tunnel: [_ w318] -> w313
            event Timeout {
              n132 = event-data() -> ()  [unwired: 1 in, 2 out]
            }
            event "chart_2": Mouse Down {
              n133 = event-data() -> ()  [unwired: 1 in, 7 out]
              n134 = call <vilib>:"Application Directory.vi"() -> ("Application Directory"=w331:path)
              n135 = Path To String(path=w331) -> (string=w330:string)
              n136 = Concatenate Strings(w330, "\\GUI\\Scope_V2_0.vi" ("名称或相对路径")) -> (w328:string)
              n137 = String To Path(string=w328) -> (path=w332:path)
              n138 = Open VI Reference(vi path=w332, options=8 ("选项")) -> (vi reference=w327:refnum<vi>, error out=w326:errorcluster)  [unwired: 4 in]
              n139 = invoke class="VI" method="FP.Open"(reference=w327, error in=w326, "Activate"=TRUE ("激活？"), "State"=T2."Standard" ("州")) -> (reference out=w323:refnum<vi>, error out=w322:errorcluster)  [unwired: 1 in, 3 out]
              n140 = invoke class="VI" method="Run VI"(reference=w323, error in=w322, "Wait until done"=FALSE ("结束前等待"), "Auto Dispose Ref"=TRUE ("自动销毁引用")) -> (reference out=w319:refnum<vi>, error out=w318:errorcluster)  [unwired: 1 in, 3 out]
            }
          }
          n141 = local read "2nd_OnOrOff"() -> (w315:bool)
          n142 = case shown="真" w315 {
            tunnel: w314 -> [_ w316]
            tunnel: w313 -> [_ w317]
            frame False {
            }
            frame True {
              n143 = Close Reference(reference=w316, error in (no error)=w317) -> ()  [unwired: 1 out]
            }
          }
        }
        n144 = while {
          tunnel: w309 -> [w348]
          tunnel: w308 -> [w347]
          tunnel: [w346] -> w312
          tunnel: [w345] -> w311
          shift-right: [w343] -> _
          shift-left: "写指令_2" -> [w344]
          tunnel: w307 -> [w342]
          tunnel: w306 -> [w341]
          tunnel: w305 -> [w339]
          tunnel: w304 -> [w338]
          stop <- w334 stop-if-true
          n145 = stacked-sequence {
            seq-local: [w362 _ _] -> [_ w402 _]
            seq-local: [w361 _ _] -> [_ w401 _]
            seq-local: [w358 _ _] -> [_ w405 _]
            seq-local: [w349 _ _] -> [_ w389 _]
            seq-local: [w350 _ _] -> [_ w399 _]
            seq-local: [_ w404 _] -> [_ _ w475]
            seq-local: [_ w403 _] -> [_ _ w474]
            seq-local: [_ w400 _] -> [_ _ w465]
            seq-local: [_ w399 _] -> [_ _ w463]
            seq-local: [_ w398 _] -> [_ _ w461]
            seq-local: [_ w393 _] -> [_ _ w454]
            seq-local: [_ w389 _] -> [_ _ w470]
            tunnel: w348 -> [w354 _ _]
            tunnel: w347 -> [w353 _ _]
            tunnel: w344 -> [w360 _ _]
            tunnel: [_ _ w478] -> w346
            tunnel: [_ _ w477] -> w345
            tunnel: [_ _ w469] -> w343
            tunnel: w342 -> [_ _ w467]
            tunnel: w341 -> [_ _ w466]
            tunnel: [_ _ w462] -> w340
            tunnel: w339 -> [_ _ w460]
            tunnel: w338 -> [_ _ w459]
            tunnel: [_ _ w454] -> w335
            frame #0 {
              n146 = VISA Flush I/O Buffer(VISA resource name=w354, error in (no error)=w353) -> (VISA resource name out=w351:refnum<visa-resource-name>, error out=w352:errorcluster)  [unwired: 1 in]
              n147 = case shown="真" w360 {
                tunnel: w354 -> [w376 _]
                tunnel: w353 -> [w375 _]
                tunnel: [w376 w384] -> w362
                tunnel: [w375 w383] -> w361
                tunnel: w352 -> [_ w378]
                tunnel: w351 -> [_ w377]
                frame False {
                }
                frame True {
                  n148 = local read "mu08SendCmd_2"() -> (w380:u8)
                  n149 = call "SendCmd.vi"("索引 (行)"=w380) -> ("字符串"=w382:string)  [unwired: 1 in]
                  "命令_2" <- w382
                  n150 = Equal?(x=w380, y=u8 3) -> (x = y?=w379:bool)
                  n151 = case shown="真" w379 {
                    frame False {
                    }
                    frame True {
                      n152 = case shown="真" "mbfUartClearOne 2" {
                        frame False {
                        }
                        frame True {
                          n153 = local write "mbfUartClearOne 2"(TRUE ("mbfUartClearOne")) -> ()
                        }
                      }
                    }
                  }
                  n154 = VISA Write(VISA resource name=w377, write buffer=w382, error in (no error)=w378) -> (VISA resource name out=w384:refnum<visa-resource-name>, error out=w383:errorcluster)  [unwired: 1 out]
                }
              }
              n155 = local read "mu08SendCmd_2"() -> (w357:u8)
              n156 = local read "CmdNumCount 2"() -> (w359:u8)
              n157 = Equal?(x=w357, y=u8 3) -> (x = y?=w355:bool)
              n158 = case shown="真" w355 {
                frame False {
                  n159 = local write "mbfDealData 2"(FALSE ("mbfDealData")) -> ()
                }
                frame True {
                  n160 = local write "mbfDealData 2"(TRUE ("mbfDealData")) -> ()
                }
              }
              n161 = case shown="3" w357 {
                tunnel: [w365 w368 w371 w374] -> w349
                frame 0, Default {
                  n162 = Multiply(x=10, y=2) -> (x*y=w365:i32)
                }
                frame 1 {
                  n163 = Multiply(x=119, y=2) -> (x*y=w368:i32)
                }
                frame 2 {
                  n164 = Multiply(x=30, y=2) -> (x*y=w371:i32)
                }
                frame 3 {
                  n165 = local read "缓冲区数据_2"() -> (w374:u32)
                }
              }
              n166 = Increment(x=w359) -> (x+1=w358:u8)
              n167 = local write "CmdNumCount 2"(w358) -> ()
              n168 = Tick Count (ms)() -> (millisecond timer value=w350:u32)
            }
            frame #1 {
              n169 = local read "mu08ArrayDatasSize_2"() -> (w392:u16)
              n170 = local read "mu16ArrayBuf0_2"() -> (w397:u16)
              n171 = Wait (ms)(milliseconds to wait=u32 400 ("等待时间（毫秒）")) -> ()  [unwired: 1 out]
              n172 = Multiply(x=w392, y=u8 2) -> (x*y=w390:u16)
              n173 = local read "mbfDealData 2"() -> (w396:bool)
              n174 = call "WWorWD.vi"("strModelChoice"="strModelChoice_2") -> ("WWorWD"=w387:bool)  [unwired: 9 in, 1 out]
              n175 = Equal?(x=w390, y=w397) -> (x = y?=w395:bool)
              n176 = And(x=w395, y=w396) -> (x .and. y?=w394:bool)
              n177 = case shown="真" w394 {
                selector: w394 -> [_ w413]
                tunnel: [w410 w431] -> w400
                tunnel: [w410 w426] -> w398
                tunnel: [FALSE w418] -> w393
                tunnel: w387 -> [_ w414]
                frame False {
                  w410 = string[] []
                }
                frame True {
                  w422 = u32 0 ("y")
                  # "TotalRemainTime = 0\n&& StepRemainTime = 0"
                  n178 = local read "mu08ArrayDatas_2"() -> (w417:u8[])
                  n179 = case shown="真" w414 {
                    tunnel: [w439 w445] -> w411
                    tunnel: [w438 w444] -> w412
                    tunnel: w417 -> [w437 w443]
                    tunnel: [18 ("索引") 20 ("索引")] -> w416
                    tunnel: [19 ("索引") 21 ("索引")] -> w415
                    tunnel: w413 -> [w434 w440]
                    frame False {
                      # "WW"
                      n180 = call "DealData.vi"("mbfDealData"=w434, "ArrayIn"=w437) -> ("mu08BufSize"=w438:u8, "Result"=w439:string[])
                    }
                    frame True {
                      # "WD"
                      n181 = call "WD_DealData.vi"("mbfDealData"=w440, "ArrayIn"=w443) -> ("ResultArrayOut"=w445:string[], "mu08BufSize"=w444:u8)
                    }
                  }
                  "mu08BufSize_2" <- w412
                  n182 = global write "strGlobalVariable.vi" "strResultArrayOut_2nd"(w411) -> ()
                  n183 = property on="strResultArrayOut 2" class="Arr (严格)"("Value"=w411) -> ()  [unwired: 2 in, 2 out]
                  n184 = call "GetDataFromString.vi"("strArrayIn"=w411) -> ("strArrayBuf"=w425:string[], "mu32ArrayOut"=w424:u32[])
                  n185 = Index Array(array=w424, index #1=w416, index #2=w415) -> (element #1=w423:u32, element #2=w421:u32)
                  n186 = Equal?(x=w423, y=w422) -> (x = y?=w420:bool)
                  n187 = Equal?(x=w422, y=w421) -> (x = y?=w419:bool)
                  n188 = Get Date/Time String(want seconds? (F)=TRUE ("需要秒？(F)")) -> (time string=w432:string)  [unwired: 2 in, 1 out]
                  n189 = Get Date/Time String(want seconds? (F)=TRUE ("需要秒？(F)")) -> (time string=w428:string)  [unwired: 2 in, 1 out]
                  n190 = And(x=w420, y=w419) -> (x .and. y?=w418:bool)
                  n191 = Insert Into Array(array=w411, index=0 ("索引"), new element=w432) -> (w431:string[])
                  n192 = Insert Into Array(array=w425, index=0 ("索引"), new element=w428) -> (w426:string[])
                }
              }
              n193 = Greater?(x=w405, y=u8 4) -> (0:w406:bool)
              n194 = case shown="真" w406 {
                tunnel: [w447 w451] -> w404
                tunnel: [w446 w450] -> w403
                tunnel: w402 -> [w447 w451]
                tunnel: w401 -> [w446 w450]
                frame False {
                  n195 = local write "写指令_2"(FALSE ("写指令")) -> ()
                }
                frame True {
                  n196 = local write "mu08SendCmd_2"(u8 3 ("mu08SendCmd")) -> ()
                  n197 = local write "CmdNumCount 2"(u8 0 ("CmdNumCount")) -> ()
                  n198 = local write "写指令_2"(TRUE ("写指令")) -> ()
                }
              }
            }
            frame #2 {
              n199 = property class="Instr"(reference=w475, error in=w474) -> (reference out=w480:refnum<visa-resource-name>, error out=w479:errorcluster, "Bytes at Port"=w457:u32)
              "缓冲区数据_2" <- w457
              n200 = VISA Read(VISA resource name=w480, byte count=w470, error in (no error)=w479) -> (VISA resource name out=w478:refnum<visa-resource-name>, read buffer=w476:string, error out=w477:errorcluster)  [unwired: 1 out]
              n201 = Greater?(x=w457, y=250) -> (0:w456:bool)
              n202 = local read "mu08SendCmd_2"() -> (w473:u8)
              n203 = case shown="真" w456 {
                tunnel: w467 -> [_ w491]
                tunnel: w466 -> [_ w490]
                tunnel: w465 -> [_ w489]
                tunnel: w461 -> [_ w488]
                tunnel: w460 -> [_ w485]
                tunnel: w459 -> [_ w484]
                frame False {
                }
                frame True {
                  n204 = Array To Spreadsheet String(array=w489, 3:"%s" ("格式字符串")) -> (spreadsheet string=w493:string)  [unwired: 1 in]
                  n205 = Array To Spreadsheet String(array=w488, 3:"%s" ("格式字符串")) -> (spreadsheet string=w486:string)  [unwired: 1 in]
                  n206 = Write to Text File(file (use dialog)=w491, text=w493, error in=w490) -> ()  [unwired: 1 in, 3 out]
                  n207 = Write to Text File(file (use dialog)=w484, text=w486, error in=w485) -> ()  [unwired: 1 in, 3 out]
                }
              }
              n208 = String To Byte Array(string=w476) -> (unsigned byte array=w455:u8[])
              "mu08ArrayBuf0 2" <- w455
              n209 = case shown="真" w456 {
                tunnel: w455 -> [_ w482]
                frame False {
                }
                frame True {
                  n210 = call "SearchData.vi"("ArrayIn"=w482) -> ("ArrayOut"=w481:u8[])  [unwired: 2 out]
                  "mu08ArrayDatas_2" <- w481
                  n211 = Array Size(array=w481) -> (size(s)=→"mu08ArrayDatasSize_2":i32)
                }
              }
              n212 = Array Size(array=w455) -> (size(s)=→"mu16ArrayBuf0_2":i32)
              n213 = Greater Or Equal?(x=w473, y=u8 4) -> (x >= y?=w471:bool)
              n214 = case shown="假" w471 {
                frame False {
                }
                frame True {
                  n215 = local write "mu08SendCmd_2"(u8 0 ("Cmd值")) -> ()
                }
              }
              n216 = local read "写指令_2"() -> (w469:bool)
              n217 = Tick Count (ms)() -> (millisecond timer value=w464:u32)
              n218 = Subtract(x=w464, y=w463) -> (x-y=w462:u32)
            }
          }
          "Time_2" <- w340
          n219 = local read "Start_2"() -> (w337:bool)
          n220 = Not(x=w337) -> (.not. x?=w336:bool)
          n221 = Or(x=w336, y=w335) -> (x .or. y?=w334:bool)
          "2nd_OnOrOff" <- w334
        }
        n222 = VISA Close(VISA resource name=w312, error in (no error)=w311) -> ()  [unwired: 1 out]
      }
    }
  }
  n223 = while {
    stop <- FALSE stop-if-true
    w509 = u16 10 items=["1.0"=10, "1.5"=15, "2.0"=20] ("stop bits (10: 1 bit)")
    n224 = call <vilib>:"Application Directory.vi"() -> ("Application Directory"=w499:path)
    n225 = Path To String(path=w499) -> (string=w498:string)
    n226 = Concatenate Strings(w498, "\\TmpDataSave\\ReceiveStrData3.xls" ("字符串")) -> (w496:string)
    n227 = String To Path(string=w496) -> (path=w502:path)
    n228 = call-poly "VISA Configure Serial Port"("VISA resource name"="3号机端口", "baud rate (9600)"=u32 9600, "data bits (8)"=u16 8, "parity (0:none)"=enum16{"None", "Odd", "Even", "Mark", "Space"}."Even", "stop bits (10: 1 bit)"=w509) -> ("VISA resource name out"=w508:refnum<visa-resource-name>, "error out"=w507:errorcluster)  [unwired: 9 in]
    n229 = VISA Flush I/O Buffer(VISA resource name=w508, error in (no error)=w507) -> (VISA resource name out=w506:refnum<visa-resource-name>, error out=w505:errorcluster)  [unwired: 1 in]
    n230 = Open/Create/Replace File(file path (use dialog)=w502, operation (0:open)=T1."open or create" ("操作(0:open)"), access (0:read/write)=enum16{"read/write", "read-only", "write-only"}."read/write" ("权限(0:read/write)")) -> (refnum out=w501:refnum<file>, error out=w500:errorcluster)  [unwired: 3 in, 1 out]
    n231 = flat-sequence {
      tunnel: w500 -> [w540]
      tunnel: w501 -> [w541]
      tunnel: w505 -> [w542]
      tunnel: w506 -> [w543]
      tunnel: [w543] -> w525
      tunnel: [w542] -> w524
      tunnel: [w541] -> w523
      tunnel: [w540] -> w522
      tunnel: [w527] -> w521
      tunnel: [w528] -> w520
      tunnel: [w549] -> w519
      tunnel: [w548] -> w518
      tunnel: [w547] -> w517
      tunnel: [w546] -> w516
      tunnel: [w545] -> w515
      tunnel: [w544] -> w514
      tunnel: w525 -> [w549]
      tunnel: w524 -> [w548]
      tunnel: w523 -> [w547]
      tunnel: w522 -> [w546]
      tunnel: w521 -> [w545]
      tunnel: w520 -> [w544]
      tunnel: w519 -> [w556]
      tunnel: w518 -> [w555]
      tunnel: w517 -> [w554]
      tunnel: w516 -> [w553]
      tunnel: w515 -> [w552]
      tunnel: w514 -> [w551]
      frame #0 {
        n232 = local write "mu08SendCmd_2 2"(u8 0 ("Cmd值")) -> ()
        n233 = local write "写指令_3"(TRUE ("写指令")) -> ()
        n234 = call <vilib>:"Application Directory.vi"() -> ("Application Directory"=w532:path)
        n235 = local write "Start_3"(FALSE ("Start_3")) -> ()
        n236 = Path To String(path=w532) -> (string=w533:string)
        n237 = Concatenate Strings(w533, "\\TmpDataSave\\ReceiveNumData3.xls" ("字符串")) -> (w535:string)
        n238 = String To Path(string=w535) -> (path=w531:path)
        n239 = Open/Create/Replace File(file path (use dialog)=w531, operation (0:open)=T1."open or create" ("操作(0:open)"), access (0:read/write)=enum16{"read/write", "read-only", "write-only"}."read/write" ("权限(0:read/write)")) -> (refnum out=w528:refnum<file>, error out=w527:errorcluster)  [unwired: 3 in, 1 out]
        "mu08SendCmd_2 2" <- u8 0 ("mu08SendCmd")
        "mbfDealData_3" <- FALSE ("mbfDealData")
      }
      frame #1 {
        n240 = while {
          stop <- "Start_3" stop-if-true
        }
      }
      frame #2 {
        n241 = while {
          stop <- w560 stop-if-true
          n242 = event shown="[1] \"chart_3\": 鼠标按下" {
            selector: _ -> [_ _]
            dyn-events: _ -> [_ _]
            timeout: _ -> [_ _]
            tunnel: [_ w566] -> w562
            tunnel: [_ w565] -> w561
            event Timeout {
              n243 = event-data() -> ()  [unwired: 1 in, 2 out]
            }
            event "chart_3": Mouse Down {
              n244 = event-data() -> ()  [unwired: 1 in, 7 out]
              n245 = call <vilib>:"Application Directory.vi"() -> ("Application Directory"=w578:path)
              n246 = Path To String(path=w578) -> (string=w577:string)
              n247 = Concatenate Strings(w577, "\\GUI\\Scope_V3_0.vi" ("名称或相对路径")) -> (w575:string)
              n248 = String To Path(string=w575) -> (path=w579:path)
              n249 = Open VI Reference(vi path=w579, options=8 ("选项")) -> (vi reference=w574:refnum<vi>, error out=w573:errorcluster)  [unwired: 4 in]
              n250 = invoke class="VI" method="FP.Open"(reference=w574, error in=w573, "Activate"=TRUE ("激活？"), "State"=T2."Standard" ("州")) -> (reference out=w570:refnum<vi>, error out=w569:errorcluster)  [unwired: 1 in, 3 out]
              n251 = invoke class="VI" method="Run VI"(reference=w570, error in=w569, "Wait until done"=FALSE ("结束前等待"), "Auto Dispose Ref"=TRUE ("自动销毁引用")) -> (reference out=w566:refnum<vi>, error out=w565:errorcluster)  [unwired: 1 in, 3 out]
            }
          }
          n252 = local read "3rd_OnorOff"() -> (w560:bool)
          n253 = case shown="真" w560 {
            tunnel: w562 -> [_ w563]
            tunnel: w561 -> [_ w564]
            frame False {
            }
            frame True {
              n254 = Close Reference(reference=w563, error in (no error)=w564) -> ()  [unwired: 1 out]
            }
          }
        }
        n255 = while {
          tunnel: w556 -> [w595]
          tunnel: w555 -> [w594]
          tunnel: [w593] -> w559
          tunnel: [w592] -> w558
          shift-right: [w590] -> _
          shift-left: "写指令_3" -> [w591]
          tunnel: w554 -> [w589]
          tunnel: w553 -> [w588]
          tunnel: w552 -> [w586]
          tunnel: w551 -> [w585]
          stop <- w582 stop-if-true
          n256 = stacked-sequence {
            seq-local: [w609 _ _] -> [_ w649 _]
            seq-local: [w608 _ _] -> [_ w648 _]
            seq-local: [w605 _ _] -> [_ w652 _]
            seq-local: [w596 _ _] -> [_ w636 _]
            seq-local: [w597 _ _] -> [_ w646 _]
            seq-local: [_ w651 _] -> [_ _ w722]
            seq-local: [_ w650 _] -> [_ _ w721]
            seq-local: [_ w647 _] -> [_ _ w712]
            seq-local: [_ w646 _] -> [_ _ w710]
            seq-local: [_ w645 _] -> [_ _ w708]
            seq-local: [_ w640 _] -> [_ _ w701]
            seq-local: [_ w636 _] -> [_ _ w717]
            tunnel: w595 -> [w601 _ _]
            tunnel: w594 -> [w600 _ _]
            tunnel: w591 -> [w607 _ _]
            tunnel: [_ _ w725] -> w593
            tunnel: [_ _ w724] -> w592
            tunnel: [_ _ w716] -> w590
            tunnel: w589 -> [_ _ w714]
            tunnel: w588 -> [_ _ w713]
            tunnel: [_ _ w709] -> w587
            tunnel: w586 -> [_ _ w707]
            tunnel: w585 -> [_ _ w706]
            tunnel: [_ _ w701] -> w581
            frame #0 {
              n257 = VISA Flush I/O Buffer(VISA resource name=w601, error in (no error)=w600) -> (VISA resource name out=w598:refnum<visa-resource-name>, error out=w599:errorcluster)  [unwired: 1 in]
              n258 = case shown="真" w607 {
                tunnel: w601 -> [w623 _]
                tunnel: w600 -> [w622 _]
                tunnel: [w623 w631] -> w609
                tunnel: [w622 w630] -> w608
                tunnel: w599 -> [_ w625]
                tunnel: w598 -> [_ w624]
                frame False {
                }
                frame True {
                  n259 = local read "mu08SendCmd_2 2"() -> (w627:u8)
                  n260 = call "SendCmd.vi"("索引 (行)"=w627) -> ("字符串"=w629:string)  [unwired: 1 in]
                  "命令_3" <- w629
                  n261 = Equal?(x=w627, y=u8 3) -> (x = y?=w626:bool)
                  n262 = case shown="真" w626 {
                    frame False {
                    }
                    frame True {
                      n263 = case shown="真" "mbfUartClearOne_3" {
                        frame False {
                        }
                        frame True {
                          n264 = local write "mbfUartClearOne_3"(TRUE ("mbfUartClearOne")) -> ()
                        }
                      }
                    }
                  }
                  n265 = VISA Write(VISA resource name=w624, write buffer=w629, error in (no error)=w625) -> (VISA resource name out=w631:refnum<visa-resource-name>, error out=w630:errorcluster)  [unwired: 1 out]
                }
              }
              n266 = local read "mu08SendCmd_2 2"() -> (w604:u8)
              n267 = local read "CmdNumCount_3"() -> (w606:u8)
              n268 = Equal?(x=w604, y=u8 3) -> (x = y?=w602:bool)
              n269 = case shown="真" w602 {
                frame False {
                  n270 = local write "mbfDealData_3"(FALSE ("mbfDealData")) -> ()
                }
                frame True {
                  n271 = local write "mbfDealData_3"(TRUE ("mbfDealData")) -> ()
                }
              }
              n272 = case shown="3" w604 {
                tunnel: [w612 w615 w618 w621] -> w596
                frame 0, Default {
                  n273 = Multiply(x=10, y=2) -> (x*y=w612:i32)
                }
                frame 1 {
                  n274 = Multiply(x=119, y=2) -> (x*y=w615:i32)
                }
                frame 2 {
                  n275 = Multiply(x=30, y=2) -> (x*y=w618:i32)
                }
                frame 3 {
                  n276 = local read "缓冲区数据_3"() -> (w621:u32)
                }
              }
              n277 = Increment(x=w606) -> (x+1=w605:u8)
              n278 = local write "CmdNumCount_3"(w605) -> ()
              n279 = Tick Count (ms)() -> (millisecond timer value=w597:u32)
            }
            frame #1 {
              n280 = local read "mu08ArrayDatasSize_3"() -> (w639:u16)
              n281 = local read "mu16ArrayBuf0_3"() -> (w644:u16)
              n282 = Wait (ms)(milliseconds to wait=u32 400 ("等待时间（毫秒）")) -> ()  [unwired: 1 out]
              n283 = Multiply(x=w639, y=u8 2) -> (x*y=w637:u16)
              n284 = local read "mbfDealData_3"() -> (w643:bool)
              n285 = call "WWorWD.vi"("strModelChoice"="strModelChoice 2") -> ("WWorWD"=w634:bool)  [unwired: 9 in, 1 out]
              n286 = Equal?(x=w637, y=w644) -> (x = y?=w642:bool)
              n287 = And(x=w642, y=w643) -> (x .and. y?=w641:bool)
              n288 = case shown="真" w641 {
                selector: w641 -> [_ w660]
                tunnel: [w657 w678] -> w647
                tunnel: [w657 w673] -> w645
                tunnel: [FALSE w665] -> w640
                tunnel: w634 -> [_ w661]
                frame False {
                  w657 = string[] []
                }
                frame True {
                  w669 = u32 0 ("y")
                  # "TotalRemainTime = 0\n&& StepRemainTime = 0"
                  n289 = local read "mu08ArrayDatas_3"() -> (w664:u8[])
                  n290 = case shown="真" w661 {
                    tunnel: [w686 w692] -> w658
                    tunnel: [w685 w691] -> w659
                    tunnel: w664 -> [w684 w690]
                    tunnel: [18 ("索引") 20 ("索引")] -> w663
                    tunnel: [19 ("索引") 21 ("索引")] -> w662
                    tunnel: w660 -> [w681 w687]
                    frame False {
                      # "WW"
                      n291 = call "DealData.vi"("mbfDealData"=w681, "ArrayIn"=w684) -> ("mu08BufSize"=w685:u8, "Result"=w686:string[])
                    }
                    frame True {
                      # "WD"
                      n292 = call "WD_DealData.vi"("mbfDealData"=w687, "ArrayIn"=w690) -> ("ResultArrayOut"=w692:string[], "mu08BufSize"=w691:u8)
                    }
                  }
                  "mu08BufSize_3" <- w659
                  n293 = global write "strGlobalVariable.vi" "strResultArrayOut_3rd"(w658) -> ()
                  n294 = property on="strResultArrayOut_3" class="Arr (严格)"("Value"=w658) -> ()  [unwired: 2 in, 2 out]
                  n295 = call "GetDataFromString.vi"("strArrayIn"=w658) -> ("strArrayBuf"=w672:string[], "mu32ArrayOut"=w671:u32[])
                  n296 = Index Array(array=w671, index #1=w663, index #2=w662) -> (element #1=w670:u32, element #2=w668:u32)
                  n297 = Equal?(x=w670, y=w669) -> (x = y?=w667:bool)
                  n298 = Equal?(x=w669, y=w668) -> (x = y?=w666:bool)
                  n299 = Get Date/Time String(want seconds? (F)=TRUE ("需要秒？(F)")) -> (time string=w679:string)  [unwired: 2 in, 1 out]
                  n300 = Get Date/Time String(want seconds? (F)=TRUE ("需要秒？(F)")) -> (time string=w675:string)  [unwired: 2 in, 1 out]
                  n301 = And(x=w667, y=w666) -> (x .and. y?=w665:bool)
                  n302 = Insert Into Array(array=w658, index=0 ("索引"), new element=w679) -> (w678:string[])
                  n303 = Insert Into Array(array=w672, index=0 ("索引"), new element=w675) -> (w673:string[])
                }
              }
              n304 = Greater?(x=w652, y=u8 4) -> (0:w653:bool)
              n305 = case shown="真" w653 {
                tunnel: [w694 w698] -> w651
                tunnel: [w693 w697] -> w650
                tunnel: w649 -> [w694 w698]
                tunnel: w648 -> [w693 w697]
                frame False {
                  n306 = local write "写指令_3"(FALSE ("写指令")) -> ()
                }
                frame True {
                  n307 = local write "mu08SendCmd_2 2"(u8 3 ("mu08SendCmd")) -> ()
                  n308 = local write "CmdNumCount_3"(u8 0 ("CmdNumCount")) -> ()
                  n309 = local write "写指令_3"(TRUE ("写指令")) -> ()
                }
              }
            }
            frame #2 {
              n310 = property class="Instr"(reference=w722, error in=w721) -> (reference out=w727:refnum<visa-resource-name>, error out=w726:errorcluster, "Bytes at Port"=w704:u32)
              "缓冲区数据_3" <- w704
              n311 = VISA Read(VISA resource name=w727, byte count=w717, error in (no error)=w726) -> (VISA resource name out=w725:refnum<visa-resource-name>, read buffer=w723:string, error out=w724:errorcluster)  [unwired: 1 out]
              n312 = Greater?(x=w704, y=250) -> (0:w703:bool)
              n313 = local read "mu08SendCmd_2 2"() -> (w720:u8)
              n314 = case shown="真" w703 {
                tunnel: w714 -> [_ w738]
                tunnel: w713 -> [_ w737]
                tunnel: w712 -> [_ w736]
                tunnel: w708 -> [_ w735]
                tunnel: w707 -> [_ w732]
                tunnel: w706 -> [_ w731]
                frame False {
                }
                frame True {
                  n315 = Array To Spreadsheet String(array=w736, 3:"%s" ("格式字符串")) -> (spreadsheet string=w740:string)  [unwired: 1 in]
                  n316 = Array To Spreadsheet String(array=w735, 3:"%s" ("格式字符串")) -> (spreadsheet string=w733:string)  [unwired: 1 in]
                  n317 = Write to Text File(file (use dialog)=w738, text=w740, error in=w737) -> ()  [unwired: 1 in, 3 out]
                  n318 = Write to Text File(file (use dialog)=w731, text=w733, error in=w732) -> ()  [unwired: 1 in, 3 out]
                }
              }
              n319 = String To Byte Array(string=w723) -> (unsigned byte array=w702:u8[])
              "mu08ArrayBuf0_3" <- w702
              n320 = case shown="真" w703 {
                tunnel: w702 -> [_ w729]
                frame False {
                }
                frame True {
                  n321 = call "SearchData.vi"("ArrayIn"=w729) -> ("ArrayOut"=w728:u8[])  [unwired: 2 out]
                  "mu08ArrayDatas_3" <- w728
                  n322 = Array Size(array=w728) -> (size(s)=→"mu08ArrayDatasSize_3":i32)
                }
              }
              n323 = Array Size(array=w702) -> (size(s)=→"mu16ArrayBuf0_3":i32)
              n324 = Greater Or Equal?(x=w720, y=u8 4) -> (x >= y?=w718:bool)
              n325 = case shown="假" w718 {
                frame False {
                }
                frame True {
                  n326 = local write "mu08SendCmd_2 2"(u8 0 ("Cmd值")) -> ()
                }
              }
              n327 = local read "写指令_3"() -> (w716:bool)
              n328 = Tick Count (ms)() -> (millisecond timer value=w711:u32)
              n329 = Subtract(x=w711, y=w710) -> (x-y=w709:u32)
            }
          }
          "Time_3" <- w587
          n330 = local read "Start_3"() -> (w584:bool)
          n331 = Not(x=w584) -> (.not. x?=w583:bool)
          n332 = Or(x=w583, y=w581) -> (x .or. y?=w582:bool)
          "3rd_OnorOff" <- w582
        }
        n333 = VISA Close(VISA resource name=w559, error in (no error)=w558) -> ()  [unwired: 1 out]
      }
    }
  }
  n334 = while {
    stop <- FALSE stop-if-true
    w756 = u16 10 items=["1.0"=10, "1.5"=15, "2.0"=20] ("stop bits (10: 1 bit)")
    n335 = call <vilib>:"Application Directory.vi"() -> ("Application Directory"=w746:path)
    n336 = Path To String(path=w746) -> (string=w745:string)
    n337 = call-poly "VISA Configure Serial Port"("VISA resource name"="1号机端口", "baud rate (9600)"=u32 9600, "data bits (8)"=u16 8, "parity (0:none)"=enum16{"None", "Odd", "Even", "Mark", "Space"}."Even", "stop bits (10: 1 bit)"=w756) -> ("VISA resource name out"=w755:refnum<visa-resource-name>, "error out"=w754:errorcluster)  [unwired: 9 in]
    n338 = Concatenate Strings(w745, "\\TmpDataSave\\ReceiveStrData.xls" ("字符串")) -> (w743:string)
    n339 = String To Path(string=w743) -> (path=w749:path)
    n340 = VISA Flush I/O Buffer(VISA resource name=w755, error in (no error)=w754) -> (VISA resource name out=w753:refnum<visa-resource-name>, error out=w752:errorcluster)  [unwired: 1 in]
    n341 = Open/Create/Replace File(file path (use dialog)=w749, operation (0:open)=T1."open or create" ("操作(0:open)"), access (0:read/write)=enum16{"read/write", "read-only", "write-only"}."read/write" ("权限(0:read/write)")) -> (refnum out=w748:refnum<file>, error out=w747:errorcluster)  [unwired: 3 in, 1 out]
    n342 = flat-sequence {
      tunnel: w747 -> [w793]
      tunnel: w748 -> [w794]
      tunnel: w752 -> [w795]
      tunnel: w753 -> [w796]
      tunnel: [w796] -> w772
      tunnel: [w795] -> w771
      tunnel: [w794] -> w770
      tunnel: [w793] -> w769
      tunnel: [w782] -> w768
      tunnel: [w783] -> w767
      tunnel: [w802] -> w766
      tunnel: [w801] -> w765
      tunnel: [w800] -> w764
      tunnel: [w799] -> w763
      tunnel: [w798] -> w762
      tunnel: [w797] -> w761
      tunnel: w772 -> [w802]
      tunnel: w771 -> [w801]
      tunnel: w770 -> [w800]
      tunnel: w769 -> [w799]
      tunnel: w768 -> [w798]
      tunnel: w767 -> [w797]
      tunnel: w766 -> [w810]
      tunnel: w765 -> [w809]
      tunnel: w764 -> [w808]
      tunnel: w763 -> [w807]
      tunnel: w762 -> [w806]
      tunnel: w761 -> [w805]
      frame #0 {
        n343 = local write "写指令"(TRUE ("写指令")) -> ()
        n344 = shared-variable "我的电脑\\GlobalVariableList.lvlib\\mu08SendCmd_1st"(u8 0 ("mu08SendCmd_1st")) -> ()  [unwired: 1 in, 1 out]
        n345 = shared-variable "我的电脑\\GlobalVariableList.lvlib\\mu083rdCmdSendCnt_1st"(u8 0 ("mu083rdCmdSendCnt_1st")) -> ()  [unwired: 1 in, 1 out]
        n346 = call <vilib>:"Application Directory.vi"() -> ("Application Directory"=w787:path)
        n347 = property on="mu08SendCmd" class="DigNum (严格)"("Value"=u8 0 ("mu08SendCmd")) -> ()  [unwired: 2 in, 2 out]
        n348 = local write "Start"(FALSE ("Start")) -> ()
        n349 = Path To String(path=w787) -> (string=w788:string)
        n350 = Concatenate Strings(w788, "\\TmpDataSave\\ReceiveNumData.xls" ("字符串")) -> (w790:string)
        n351 = String To Path(string=w790) -> (path=w786:path)
        n352 = Open/Create/Replace File(file path (use dialog)=w786, operation (0:open)=T1."open or create" ("操作(0:open)"), access (0:read/write)=enum16{"read/write", "read-only", "write-only"}."read/write" ("权限(0:read/write)")) -> (refnum out=w783:refnum<file>, error out=w782:errorcluster)  [unwired: 3 in, 1 out]
        "mbfDealData" <- FALSE ("mbfDealData")
        "strResultArrayOut" <- string[] []
        "mbfSendStop" <- TRUE ("mbfSendStop")
        "mu08SendCountStop" <- u8 0 ("mu08SendCountStop")
        "写指令" <- TRUE ("写指令")
        "mu083rdCmdSendCount" <- u8 0 ("mu083rdCmdSendCount")
      }
      frame #1 {
        n353 = while {
          stop <- "Start" stop-if-true
        }
      }
      frame #2 {
        n354 = while {
          stop <- w815 stop-if-true
          n355 = event shown="[1] \"chart\": 鼠标按下" {
            selector: _ -> [_ _]
            dyn-events: _ -> [_ _]
            timeout: _ -> [_ _]
            tunnel: [_ w823] -> w814
            tunnel: [_ w822] -> w813
            event Timeout {
              n356 = event-data() -> ()  [unwired: 1 in, 2 out]
            }
            event "chart": Mouse Down {
              n357 = event-data() -> ()  [unwired: 1 in, 7 out]
              n358 = property on="WWorWD" class="Bool (严格)"() -> ("Value"=w818:bool)  [unwired: 2 in, 2 out]
              n359 = case shown="假" w818 {
                tunnel: ["\\GUI\\Scope_V1_0_A.vi" ("名称或相对路径") "\\GUI\\Scope_V1_0.vi" ("名称或相对路径")] -> w819
                frame False {
                }
                frame True {
                }
              }
              n360 = call <vilib>:"Application Directory.vi"() -> ("Application Directory"=w832:path)
              n361 = Path To String(path=w832) -> (string=w831:string)
              n362 = Concatenate Strings(w831, w819) -> (w830:string)
              n363 = String To Path(string=w830) -> (path=w833:path)
              n364 = Open VI Reference(vi path=w833, options=8 ("选项")) -> (vi reference=w829:refnum<vi>, error out=w828:errorcluster)  [unwired: 4 in]
              n365 = invoke class="VI" method="FP.Open"(reference=w829, error in=w828, "Activate"=TRUE ("激活？"), "State"=T2."Standard" ("州")) -> (reference out=w825:refnum<vi>, error out=w824:errorcluster)  [unwired: 1 in, 3 out]
              n366 = invoke class="VI" method="Run VI"(reference=w825, error in=w824, "Wait until done"=FALSE ("结束前等待"), "Auto Dispose Ref"=TRUE ("自动销毁引用")) -> (reference out=w823:refnum<vi>, error out=w822:errorcluster)  [unwired: 1 in, 3 out]
            }
          }
          n367 = local read "1st_OnorOff"() -> (w815:bool)
          n368 = case shown="真" w815 {
            tunnel: w814 -> [_ w817]
            tunnel: w813 -> [_ w816]
            frame False {
            }
            frame True {
              n369 = Close Reference(reference=w817, error in (no error)=w816) -> ()  [unwired: 1 out]
            }
          }
        }
        n370 = local read "写指令"() -> (w804:bool)
        n371 = while {
          tunnel: w810 -> [w874]
          tunnel: w809 -> [w873]
          tunnel: [w872] -> w812
          tunnel: [w871] -> w811
          shift-right: [w869] -> _
          shift-left: w804 -> [w870]
          tunnel: w808 -> [w868]
          tunnel: w807 -> [w867]
          tunnel: w806 -> [w865]
          tunnel: w805 -> [w864]
          stop <- FALSE stop-if-true
          n372 = flat-sequence {
            tunnel: w874 -> [w894]
            tunnel: w873 -> [w893]
            tunnel: w870 -> [w898]
            tunnel: w868 -> [w880]
            tunnel: w867 -> [w890]
            tunnel: [w890] -> w859
            tunnel: w865 -> [w879]
            tunnel: w864 -> [w889]
            tunnel: [w889] -> w858
            tunnel: [w877] -> w857
            tunnel: [w896] -> w856
            tunnel: [w881] -> w855
            tunnel: [w876] -> w854
            tunnel: [w883] -> w842
            tunnel: [w880] -> w840
            tunnel: [w879] -> w839
            tunnel: [w878] -> w838
            tunnel: [w875] -> w837
            tunnel: [w937] -> w853
            tunnel: w859 -> [w936]
            tunnel: [w936] -> w852
            tunnel: [w927] -> w851
            tunnel: w858 -> [w935]
            tunnel: [w935] -> w850
            tunnel: w857 -> [w951]
            tunnel: w856 -> [w954]
            tunnel: w855 -> [w933]
            tunnel: w854 -> [w934]
            tunnel: [w953] -> w849
            tunnel: [w952] -> w848
            tunnel: [w949] -> w847
            tunnel: [w934] -> w846
            tunnel: [w948] -> w845
            tunnel: [w943] -> w844
            tunnel: [w933] -> w843
            tunnel: w842 -> [w928]
            tunnel: w840 -> [w937]
            tunnel: w839 -> [w927]
            tunnel: w838 -> [w950]
            tunnel: w837 -> [w930]
            tunnel: [w1038] -> w872
            tunnel: [w1037] -> w871
            tunnel: [w1029] -> w869
            tunnel: w853 -> [w1028]
            tunnel: w852 -> [w1027]
            tunnel: [w1023] -> w866
            tunnel: w851 -> [w1021]
            tunnel: w850 -> [w1020]
            tunnel: [w1015] -> w863
            tunnel: w849 -> [w1035]
            tunnel: w848 -> [w1034]
            tunnel: w847 -> [w1026]
            tunnel: w846 -> [w1024]
            tunnel: w845 -> [w1022]
            tunnel: w844 -> [w1015]
            tunnel: w843 -> [w1030]
            frame #0 {
              n373 = VISA Flush I/O Buffer(VISA resource name=w894, error in (no error)=w893) -> (VISA resource name out=w891:refnum<visa-resource-name>, error out=w892:errorcluster)  [unwired: 1 in]
              n374 = property on="mu08SendCmd" class="DigNum (严格)"() -> ("Value"=w883:u8)  [unwired: 2 in, 2 out]
              n375 = case shown="真" w898 {
                tunnel: w894 -> [w913 _]
                tunnel: w893 -> [w912 _]
                tunnel: [w913 w924] -> w877
                tunnel: [w912 w923] -> w878
                tunnel: w892 -> [_ w921]
                tunnel: w891 -> [_ w920]
                tunnel: w883 -> [_ w915]
                frame False {
                }
                frame True {
                  n376 = Equal?(x=u8 4 ("y"), y=w915) -> (x = y?=w918:bool)
                  n377 = call "SendCmd.vi"("索引 (行)"=w915) -> ("字符串"=w914:string)  [unwired: 1 in]
                  "命令" <- w914
                  n378 = Equal?(x=w915, y=u8 3) -> (x = y?=w917:bool)
                  n379 = Or(x=w918, y=w917) -> (x .or. y?=w916:bool)
                  n380 = case shown="真" w916 {
                    frame False {
                    }
                    frame True {
                      n381 = case shown="真" "mbfUartClearOne" {
                        frame False {
                        }
                        frame True {
                          n382 = local write "mbfUartClearOne"(TRUE ("mbfUartClearOne")) -> ()
                        }
                      }
                    }
                  }
                  n383 = VISA Write(VISA resource name=w920, write buffer=w914, error in (no error)=w921) -> (VISA resource name out=w924:refnum<visa-resource-name>, error out=w923:errorcluster)  [unwired: 1 out]
                }
              }
              n384 = property on="mu08SendCountStop" class="DigNum (严格)"() -> ("Value"=w875:u8)  [unwired: 2 in, 2 out]
              n385 = Increment(x=w875) -> (x+1=w888:u8)
              n386 = property on="mu08SendCountStop" class="DigNum (严格)"("Value"=w888) -> ()  [unwired: 2 in, 2 out]
              n387 = local read "CmdNumCount"() -> (w897:u8)
              n388 = Equal?(x=w883, y=u8 4) -> (x = y?=w885:bool)
              n389 = Equal?(x=w883, y=u8 3) -> (x = y?=w886:bool)
              n390 = local read "缓冲区数据"() -> (w882:u32)
              n391 = Or(x=w886, y=w885) -> (x .or. y?=w884:bool)
              n392 = case shown="真" w884 {
                frame False {
                  n393 = local write "mbfDealData"(FALSE ("mbfDealData")) -> ()
                }
                frame True {
                  n394 = local write "mbfDealData"(TRUE ("mbfDealData")) -> ()
                }
              }
              n395 = case shown="4" w883 {
                tunnel: [w901 w904 w907 w910 w911] -> w881
                tunnel: w882 -> [_ _ _ w910 w911]
                frame 0, Default {
                  n396 = Multiply(x=10, y=2) -> (x*y=w901:i32)
                }
                frame 1 {
                  n397 = Multiply(x=119, y=2) -> (x*y=w904:i32)
                }
                frame 2 {
                  n398 = Multiply(x=30, y=2) -> (x*y=w907:i32)
                }
                frame 3 {
                }
                frame 4 {
                }
              }
              n399 = Increment(x=w897) -> (x+1=w896:u8)
              n400 = local write "CmdNumCount"(w896) -> ()
              n401 = Tick Count (ms)() -> (millisecond timer value=w876:u32)
            }
            frame #1 {
              n402 = local read "mu08ArrayDatasSize"() -> (w942:u16)
              n403 = Wait (ms)(milliseconds to wait=u32 400 ("等待时间（毫秒）")) -> ()  [unwired: 1 out]
              n404 = local read "mu16ArrayBuf0"() -> (w947:u16)
              n405 = Multiply(x=w942, y=u8 2) -> (x*y=w940:u16)
              n406 = local read "mbfDealData"() -> (w946:bool)
              n407 = call "WWorWD.vi"("strModelChoice"="strModelChoice") -> ("WWorWD"=w938:bool)  [unwired: 9 in, 1 out]
              "WWorWD" <- w938
              n408 = Equal?(x=w940, y=w947) -> (x = y?=w945:bool)
              n409 = Greater?(x=w930, y=u8 7) -> (0:w931:bool)
              n410 = And(x=w945, y=w946) -> (x .and. y?=w944:bool)
              n411 = case shown="真" w931 {
                tunnel: [u8 4 ("y") u8 100 ("y")] -> w929
                frame False {
                }
                frame True {
                  n412 = property on="mu08SendCountStop" class="DigNum (严格)"("Value"=u8 9 ("mu08SendCountStop")) -> ()  [unwired: 2 in, 2 out]
                }
              }
              n413 = case shown="真" w944 {
                selector: w944 -> [_ w965]
                tunnel: [w961 w982] -> w949
                tunnel: [w961 w977] -> w948
                tunnel: [FALSE FALSE] -> w943
                tunnel: w938 -> [_ w966]
                frame False {
                  w961 = string[] []
                }
                frame True {
                  w973 = u32 0 ("y")
                  # "TotalRemainTime = 0\n&& StepRemainTime = 0"
                  n414 = local read "mu08ArrayDatas"() -> (w969:u8[])
                  n415 = case shown="假" w966 {
                    tunnel: [w990 w991] -> w963
                    tunnel: [w989 w996] -> w964
                    tunnel: w969 -> [w988 w995]
                    tunnel: [18 ("索引") 20 ("索引")] -> w968
                    tunnel: [19 ("索引") 21 ("索引")] -> w967
                    tunnel: w965 -> [w985 w992]
                    frame False {
                      # "WW"
                      n416 = call "DealData.vi"("mbfDealData"=w985, "ArrayIn"=w988) -> ("mu08BufSize"=w989:u8, "Result"=w990:string[])
                    }
                    frame True {
                      # "WD"
                      n417 = call "WD_DealData.vi"("mbfDealData"=w992, "ArrayIn"=w995) -> ("ResultArrayOut"=w991:string[], "mu08BufSize"=w996:u8)
                    }
                  }
                  "mu08BufSize" <- w964
                  n418 = global write "strGlobalVariable.vi" "strResultArrayOut_1st"(w963) -> ()
                  n419 = property on="strResultArrayOut" class="Arr (严格)"("Value"=w963) -> ()  [unwired: 2 in, 2 out]
                  n420 = call "GetDataFromString.vi"("strArrayIn"=w963) -> ("strArrayBuf"=w976:string[], "mu32ArrayOut"=w975:u32[])
                  n421 = Index Array(array=w975, index #1=w968, index #2=w967) -> (element #1=w974:u32, element #2=w972:u32)
                  n422 = Equal?(x=w974, y=w973) -> (x = y?=w971:bool)
                  n423 = Equal?(x=w973, y=w972) -> (x = y?=w970:bool)
                  n424 = Get Date/Time String(want seconds? (F)=TRUE ("需要秒？(F)")) -> (time string=w983:string)  [unwired: 2 in, 1 out]
                  n425 = Get Date/Time String(want seconds? (F)=TRUE ("需要秒？(F)")) -> (time string=w979:string)  [unwired: 2 in, 1 out]
                  n426 = And(x=w971, y=w970) -> ()  [unwired: 1 out]
                  n427 = Insert Into Array(array=w963, index=0 ("索引"), new element=w983) -> (w982:string[])
                  n428 = Insert Into Array(array=w976, index=0 ("索引"), new element=w979) -> (w977:string[])
                }
              }
              n429 = Greater?(x=w954, y=w929) -> (0:w955:bool)
              n430 = case shown="真" w955 {
                tunnel: [w998 w1003] -> w953
                tunnel: [w997 w1002] -> w952
                tunnel: w951 -> [w998 w1003]
                tunnel: w950 -> [w997 w1002]
                tunnel: w928 -> [_ w1001]
                frame False {
                  n431 = local write "写指令"(FALSE ("写指令")) -> ()
                }
                frame True {
                  n432 = case shown="4" w1001 {
                    tunnel: [u8 3 ("mu08SendCmd") u8 3 ("mu08SendCmd") u8 3 ("mu08SendCmd") u8 4 ("mu08SendCmd") u8 4 ("mu08SendCmd")] -> w1000
                    frame 0, Default {
                    }
                    frame 1 {
                    }
                    frame 2 {
                    }
                    frame 3 {
                    }
                    frame 4 {
                    }
                  }
                  n433 = local write "CmdNumCount"(u8 0 ("CmdNumCount")) -> ()
                  n434 = local write "写指令"(TRUE ("写指令")) -> ()
                  n435 = property on="mu08SendCmd" class="DigNum (严格)"("Value"=w1000) -> ()  [unwired: 2 in, 2 out]
                }
              }
            }
            frame #2 {
              n436 = property on="mu08SendCmd" class="DigNum (严格)"() -> ("Value"=w1014:u8)  [unwired: 2 in, 2 out]
              n437 = Equal?(x=w1014, y=4) -> (x = y?=w1012:bool)
              n438 = case shown="假" w1012 {
                tunnel: [200 ("y") 200 ("y")] -> w1011
                frame False {
                }
                frame True {
                }
              }
              n439 = property class="Instr"(reference=w1035, error in=w1034) -> (reference out=w1040:refnum<visa-resource-name>, error out=w1039:errorcluster, "Bytes at Port"=w1018:u32)
              "缓冲区数据" <- w1018
              n440 = VISA Read(VISA resource name=w1040, byte count=w1030, error in (no error)=w1039) -> (VISA resource name out=w1038:refnum<visa-resource-name>, read buffer=w1036:string, error out=w1037:errorcluster)  [unwired: 1 out]
              n441 = Greater?(x=w1018, y=w1011) -> (0:w1017:bool)
              n442 = local read "mu08SendCmd"() -> (w1033:u8)
              n443 = case shown="真" w1017 {
                tunnel: w1028 -> [_ w1053]
                tunnel: w1027 -> [_ w1052]
                tunnel: w1026 -> [_ w1051]
                tunnel: w1022 -> [_ w1050]
                tunnel: w1021 -> [_ w1047]
                tunnel: w1020 -> [_ w1046]
                frame False {
                }
                frame True {
                  n444 = Array To Spreadsheet String(array=w1051, 3:"%s" ("格式字符串")) -> (spreadsheet string=w1055:string)  [unwired: 1 in]
                  n445 = Array To Spreadsheet String(array=w1050, 3:"%s" ("格式字符串")) -> (spreadsheet string=w1048:string)  [unwired: 1 in]
                  n446 = Write to Text File(file (use dialog)=w1053, text=w1055, error in=w1052) -> ()  [unwired: 1 in, 3 out]
                  n447 = Write to Text File(file (use dialog)=w1046, text=w1048, error in=w1047) -> ()  [unwired: 1 in, 3 out]
                }
              }
              n448 = String To Byte Array(string=w1036) -> (unsigned byte array=w1016:u8[])
              "mu08ArrayBuf0" <- w1016
              n449 = Array Size(array=w1016) -> (size(s)=→"mu16ArrayBuf0":i32)
              n450 = case shown="真" w1017 {
                tunnel: w1016 -> [_ w1044]
                frame False {
                }
                frame True {
                  n451 = call "SearchData.vi"("ArrayIn"=w1044) -> ("ArrayOut"=w1043:u8[])  [unwired: 2 out]
                  "mu08ArrayDatas" <- w1043
                  n452 = Array Size(array=w1043) -> (size(s)=→"mu08ArrayDatasSize":i32)
                }
              }
              n453 = Greater Or Equal?(x=w1033, y=u8 5) -> (x >= y?=w1031:bool)
              n454 = case shown="真" w1031 {
                frame False {
                }
                frame True {
                  n455 = local write "mu08SendCmd"(u8 0 ("Cmd值")) -> ()
                }
              }
              n456 = Tick Count (ms)() -> (millisecond timer value=w1025:u32)
              n457 = local read "写指令"() -> (w1029:bool)
              n458 = Subtract(x=w1025, y=w1024) -> (x-y=w1023:u32)
            }
          }
          n459 = local read "Start"() -> (w861:bool)
          n460 = Not(x=w861) -> (.not. x?=w860:bool)
          n461 = Or(x=w860, y=w863) -> (x .or. y?=→"1st_OnorOff":bool)
          "Time" <- w866
        }
        n462 = VISA Close(VISA resource name=w812, error in (no error)=w811) -> ()  [unwired: 1 out]
      }
    }
  }
